vi "app - monitor RUS scan - P1.vi"() -> ()   [LabVIEW 2014]
uses:
  complex region.ctl
  lorentzian.ctl
  circle corners.ctl
  cursor winow.ctl
  scale - offset gauge.ctl
  <vilib>/event_ctls.llb/eventvkey.ctl
  peak -- parameters -- complex fit.ctl
  wavepacket.ctl
  filter method control.ctl
  parameters -- scan monitor control.ctl
  monitor state.ctl
  peak monitor ctl.ctl
  interpolation state - real.ctl
  countdown control.ctl
  cursor window action.ctl
  plot refs -- filter related.ctl
  monitor action.ctl
  read scan file control.ctl
  ctl -- name dispatcher -- action.ctl
  Q -- check range -- i -- real - window.vi
  array -- find interval - real.vi
  next chunk - read-write freq PID file - atomic actions .vi
  Q -- check range -- i -- integer.vi
  aggregator - iii - real - atomic.vi
  switch - C.vi
  acquire cursor window data.vi
  filter - complex - four.vi
  peak -- PM find lorenzian - V2.vi
  Q - not nan -- real.vi
  array -- find index - real.vi
  array -- interpolate -- i.vi
  Q - not nan -- integer.vi
  linear interpolation - real.vi
  tale of three indices.vi
  filter -- window span logic.vi
  linear interp iiii- complex - z-omega - divide.vi
  linear interpolation iiii- complex.vi
  containing bix.vi
  peak -- guess at omega -- dzdomega.vi
  command stack.vi
  tale of three indices -- check state.vi
  linear interp iiii- complex - z-omega.vi
  line -- complex.vi
  peak -- z center from mult phase points.vi
  peak -- estimate for lorentzian.vi
  peak -- fake phase around center.vi
  peak -- get weights.vi
  peak -- four corner circle transformation logic.vi
  peak - fit phase around center - V1.vi
  <vilib>/Analysis/baseanly.llb/A x B.vi
  <vilib>/Analysis/baseanly.llb/Complex A x B.vi
  circle center from three points.vi
  <vilib>/Utility/error.llb/Clear Errors.vi
  Split file name.vi
  <vilib>/Utility/file.llb/Read From Spreadsheet File.vi
  <vilib>/Utility/file.llb/Read From Spreadsheet File (DBL).vi
  <vilib>/Utility/file.llb/Read From Spreadsheet File (string).vi
  Q regex box.vi
  <vilib>/Utility/libraryn.llb/Check if File or Folder Exists.vi
  file -- read list of lines.vi
  parse -- find first line.vi
  parse -- get list of matches -- numbers.vi
  <vilib>/Utility/file.llb/Write To Spreadsheet File (string).vi
  <vilib>/gmath/function.llb/Binomial Coefficient.vi
  monitor -- write section files.vi
  <vilib>/Analysis/Matrix/Numeric/Conversions/Array To Matrix.vi
  <vilib>/Analysis/Matrix/Numeric/Conversions/Array To Matrix - RA2.vi
  <vilib>/Analysis/baseanly.llb/Inverse Matrix.vi
  <vilib>/Analysis/baseanly.llb/Real Inverse Matrix.vi
  array - generate range.vi
  peak -- fit function -- arctan.vi
  <vilib>/gmath/NumericalOptimization/Nonlinear Curve Fit.vi
  <vilib>/gmath/NumericalOptimization/Nonlinear Curve Fit LM.vi
  filter pipe - plot staff - more - V2.vi
panel:
  in  "overwriting !!":bool
  in  "current resonance #":i32=2
  in  "overwrite (d)":enum16{"DUMP", "WORK", ""}(ring)
  in  "Tab : monitor":enum32{"main", "EDIT"}(tab)
  out "index -- main":i32[](array[numeric])=[0, 1, 2, 3, 4, 5, 6, 7, 8, 9, 10, 11, 12, 13, 14, 15, 16, 17, 18, 19, 20, 21, 22, 23, 24, 25, 26, 27, 28, 29, 30, 31, 32, 33, 34, 35, 36, 37, 38, 39, 40, 41, 42, 43, 44, 45, 46, 47, 48, 49, 50, 51, 52, 53, 54, 55, 56, 57, 58, 59, 60, 61, 62, 63, 64, 65, 66, 67, 68, 69, 70, 71, 72, 73, 74, 75, 76, 77, 78, 79, 80, 81, 82, 83, 84, 85, 86, 87, 88, 89, 90, 91, 92, 93, 94, 95, 96, 97, 98, 99]
  in  "scan monitor control":T1={"gamma acc. - min "=0.3, "gamma acc. - max"=3.0, "peak acc. fraction"=4.0, "min peak acc. window (kHz)"=0.5, "use"=enum."fraction", "abs gamma min(kHz)"=0.01, "abs gamma max(kHz)"=10.0, "# points"=10, "gamma-factor"=4.0, "interpolate"=enum."line", "init"=TRUE, "Unique peak \nparameters"=FALSE, "max peak acc. window (kHz)"=15.0, "spacing factor"=1.5, "iterate #"=1, "overwrite?"=TRUE, "write \nm files?"=TRUE, "max slope"=0.5}
  in  "monitor state":T2={"header - gamma"=[], "header - frequency"=[], "# of peaks"=6, "peaks OK"=FALSE}
  in  "autopilot":enum32{"on", "off"}(tab)=enum."off"
  in  "\"o\" timer selector":enum32{"absol", "watch"}(tab)=enum."watch"
  in  "timer \"o\"":dbl(slide)=156.2819999998901 min=-451299679.0000001 max=2129711151.0 step=0.010000000000000002 scale=0.0..320.0 scale format="%#3_3f"
  in  "timer  \"update\"":dbl(slide)=6.281999999890104 min=-451449679.0000001 max=2129711151.0 step=0.010000000000000002 scale=0.0..10.0 scale format="%#3_3f"
  in  "timer \"v\"":dbl(slide)=1.2710000000079162 min=-451454690.0 max=2129711151.0 step=0.01 scale=0.0..5.0 scale format="%#3_3f"
  in  "Temperature (K)":dbl=46.363
  in  "Magn Field (T)":dbl
  in  "Array of states":T3[](array[typedef])=[{"delta"=30.039245391659023, "gamma"=0.02588, "exp"=212.58431, "found?"=FALSE, "found"=242.623555391659, "gamma found"=8.56555840842866e-05, "init linear"=TRUE, "interpolate"=enum."line", "gamma-factor"=4.0, "slope"=0.0, "update freq?"=TRUE, "update gamma?"=FALSE, "acc factor"=4.0, "linear interpolation state"={"requested size"=10, "Array"=[0.0, 0.0, 0.0, 0.0, 0.0, 0.0, 0.0, 0.0, 0.0, 212.58431], "actual number of elements"=1}}, {"delta"=0.058120035166581374, "gamma"=0.02588, "exp"=200.03416, "found?"=FALSE, "found"=200.0922800351666, "gamma found"=0.029880221491734887, "init linear"=TRUE, "interpolate"=enum."line", "gamma-factor"=4.0, "slope"=0.0, "update freq?"=TRUE, "update gamma?"=FALSE, "acc factor"=4.0, "linear interpolation state"={"requested size"=10, "Array"=[0.0, 0.0, 0.0, 0.0, 0.0, 0.0, 0.0, 0.0, 0.0, 200.03416], "actual number of elements"=1}}, {"delta"=-414.585032797282, "gamma"=10.0, "exp"=521.21905, "found?"=FALSE, "found"=106.63401720271804, "gamma found"=859.856632431685, "init linear"=FALSE, "interpolate"=enum."line", "gamma-factor"=4.0, "slope"=0.2048099999999712, "update freq?"=TRUE, "update gamma?"=TRUE, "acc factor"=4.0, "linear interpolation state"={"requested size"=10, "Array"=[523.06234, 522.85753, 522.65272, 522.44791, 522.2431, 522.03829, 521.83348, 521.62867, 521.42386, 521.21905], "actual number of elements"=10}}, {"delta"=-82.56675261318571, "gamma"=10.0, "exp"=900.77722, "found?"=FALSE, "found"=818.2104673868143, "gamma found"=202.9884321626993, "init linear"=TRUE, "interpolate"=enum."line", "gamma-factor"=4.0, "slope"=0.0, "update freq?"=TRUE, "update gamma?"=FALSE, "acc factor"=4.0, "linear interpolation state"={"requested size"=10, "Array"=[0.0, 0.0, 0.0, 0.0, 0.0, 0.0, 0.0, 0.0, 0.0, 900.77722], "actual number of elements"=1}}, {"delta"=-2808.68343, "gamma"=0.01, "exp"=2808.68343, "found?"=FALSE, "found"=0.0, "gamma found"=0.0, "init linear"=TRUE, "interpolate"=enum."line", "gamma-factor"=2.0, "slope"=0.0, "update freq?"=TRUE, "update gamma?"=FALSE, "acc factor"=2.0, "linear interpolation state"={"requested size"=10, "Array"=[0.0, 0.0, 0.0, 0.0, 0.0, 0.0, 0.0, 0.0, 0.0, 2808.68343], "actual number of elements"=1}}, {"delta"=115.97601993996977, "gamma"=10.0, "exp"=2981.49794, "found?"=FALSE, "found"=3097.47395993997, "gamma found"=145.01354836282937, "init linear"=TRUE, "interpolate"=enum."line", "gamma-factor"=6.0, "slope"=0.0, "update freq?"=TRUE, "update gamma?"=FALSE, "acc factor"=6.0, "linear interpolation state"={"requested size"=10, "Array"=[0.0, 0.0, 0.0, 0.0, 0.0, 0.0, 0.0, 0.0, 0.0, 2981.49794], "actual number of elements"=1}}]
  in  "dump/work NEW (\"n\")":enum16{"DUMP", "WORK", ""}(ring)
  in  "NEW freq":dbl[](array[numeric])=[212.58431, 200.03416, 521.01424, 900.77722, 2808.68343, 2981.49794]
  in  "NEW gamma":dbl[](array[numeric])=[0.02588, 0.02588, 10.0, 10.0, 0.01, 10.0]
  in  "OLD gamma":dbl[](array[numeric])=[0.02588, 0.02588, 10.0, 10.0, 0.01, 10.0]
  in  "OLD freq":dbl[](array[numeric])=[212.58431, 200.03416, 521.21905, 900.77722, 2808.68343, 2981.49794]
  out "cp lorentzian":T5={"Amplitude"=0.04556963061640163, "omega(0)"=3097.47395993997, "Gamma"=145.01354836282937, "phase"=-0.8570973522961745, "Q"=21.359893574840147, "Norm  Ampl"=nan, "z (inf)"=0.0028057937941274873+0.005057236434013693i, "4corners"={"z (-pi/2)"=0.002773957390370687+0.0046139701857242825i, "z(inf)"=0.0028057937941274873+0.005057236434013693i, "z (pi/2)"=0.0023625275458380767+0.005089072837770493i, "z center"=0.0025682424681043817+0.004851521511747388i, "z(0)"=0.002330691142081276+0.004645806589481083i, "radius"=0.0003142439525883794}} {"z (inf)" format="%#9_9f"; "Q" format="%#9_9f"; "phase" format="%#9_9f"; "Gamma" format="%#9_9f"; "omega(0)" format="%#9_9f"}
  out "index":i32[](array[numeric])=[0, 1, 2, 3, 4, 5, 6, 7, 8, 9, 10, 11, 12, 13, 14, 15, 16, 17, 18, 19, 20, 21, 22, 23, 24, 25, 26, 27, 28, 29, 30, 31, 32, 33, 34, 35, 36, 37, 38, 39, 40, 41, 42, 43, 44, 45, 46, 47, 48, 49, 50, 51, 52, 53, 54, 55, 56, 57, 58, 59, 60, 61, 62, 63, 64, 65, 66, 67, 68, 69, 70, 71, 72, 73, 74, 75, 76, 77, 78, 79, 80, 81, 82, 83, 84, 85, 86, 87, 88, 89, 90, 91, 92, 93, 94, 95, 96, 97, 98, 99]
  in  "Tab : everything":T7(tab)
  in  "Tab :  Fit controls":enum32{"complex plane", "complex plane 2"}(tab)
  in  "Plot: fragment - filter":cluster{dbl[], dbl[]}[](graph)=[{array[466 elements], array[466 elements]}, {array[466 elements], array[466 elements]}, {array[466 elements], array[466 elements]}, {array[466 elements], array[466 elements]}]
  in  "scale gauge: Plot: complex plane - filter":dbl(slide)=0.001 min=0.0 max=0.3 step=1e-05 scale=0.0001..0.3 scale format="%#_2g"
  in  "Plot: complex plane - filter":cluster{dbl[], dbl[]}[](graph)=[{array[466 elements], array[466 elements]}, {array[466 elements], array[466 elements]}, {[0.009289136459626816, 0.00928889692413463, 0.009288179262995223, 0.009286986308489249, 0.009285322768663132, 0.009283195208748563, 0.00928061202525254, 0.009277583412820176, 0.0092741213240011, 0.009270239422078202, 0.0092659530271449, 0.009261279055643728, 0.009256235953604868, 0.009250843623848093, 0.009245123347435429, 0.009239097699684534, 0.009232790461074223, 0.009226226523393789, 0.009219431791506477, 0.00921243308111483, 0.009205258012931357, 0.0091979349036722, 0.009190492654303994, 0.009182960635984958, 0.009175368574150343, 0.009167746431199728, 0.009160124288249112, 0.009152532226414498, 0.009145000208095461, 0.009137557958727257, 0.0091302348494681, 0.009123059781284627, 0.009116061070892979, 0.009109266339005667, 0.009102702401325232, 0.009096395162714922, 0.009090369514964027, 0.009084649238551363, 0.009079256908794587, 0.009074213806755728, 0.009069539835254556, 0.009065253440321254, 0.009061371538398356, 0.00905790944957928, 0.009054880837146916, 0.009052297653650893, 0.009050170093736324, 0.009048506553910207, 0.009047313599404232, 0.009046595938264826, 0.00904635640277264, 0.009046595938264826, 0.009047313599404232, 0.009048506553910207, 0.009050170093736324, 0.009052297653650893, 0.009054880837146916, 0.00905790944957928, 0.009061371538398356, 0.009065253440321254, 0.009069539835254556, 0.009074213806755728, 0.009079256908794587, 0.009084649238551363, 0.009090369514964027, 0.009096395162714922, 0.009102702401325232, 0.009109266339005667, 0.009116061070892979, 0.009123059781284627, 0.0091302348494681, 0.009137557958727257, 0.009145000208095461, 0.009152532226414498, 0.009160124288249112, 0.009167746431199728, 0.009175368574150343, 0.009182960635984958, 0.009190492654303994, 0.0091979349036722, 0.009205258012931357, 0.00921243308111483, 0.009219431791506477, 0.009226226523393789, 0.009232790461074223, 0.009239097699684534, 0.009245123347435429, 0.009250843623848093, 0.009256235953604868, 0.009261279055643728, 0.0092659530271449, 0.009270239422078202, 0.0092741213240011, 0.009277583412820176, 0.00928061202525254, 0.009283195208748563, 0.009285322768663132, 0.009286986308489249, 0.009288179262995223, 0.00928889692413463], [0.002651237221672282, 0.002658859364622897, 0.002666451426457512, 0.002673983444776548, 0.002681425694144753, 0.00268874880340391, 0.002695923871587384, 0.0027029225819790313, 0.002709717313866343, 0.002716281251546778, 0.0027225884901570883, 0.002728614137907983, 0.002734334414320646, 0.002739726744077422, 0.0027447698461162827, 0.002749443817617454, 0.0027537302125507554, 0.0027576121144736536, 0.00276107420329273, 0.0027641028157250947, 0.002766685999221118, 0.002768813559135685, 0.0027704770989618035, 0.0027716700534677783, 0.002772387714607183, 0.0027726272500993698, 0.002772387714607183, 0.0027716700534677783, 0.0027704770989618035, 0.002768813559135685, 0.002766685999221118, 0.0027641028157250947, 0.00276107420329273, 0.0027576121144736536, 0.0027537302125507554, 0.002749443817617454, 0.0027447698461162827, 0.002739726744077422, 0.002734334414320646, 0.002728614137907983, 0.0027225884901570883, 0.002716281251546778, 0.002709717313866343, 0.0027029225819790313, 0.002695923871587384, 0.00268874880340391, 0.002681425694144753, 0.002673983444776548, 0.0026664514264575115, 0.002658859364622897, 0.002651237221672282, 0.002643615078721667, 0.002636023016887052, 0.002628490998568016, 0.002621048749199811, 0.0026137256399406538, 0.00260655057175718, 0.0025995518613655326, 0.002592757129478221, 0.002586193191797786, 0.0025798859531874756, 0.002573860305436581, 0.002568140029023918, 0.002562747699267142, 0.002557704597228281, 0.00255303062572711, 0.002548744230793808, 0.0025448623288709103, 0.0025414002400518335, 0.002538371627619469, 0.002535788444123446, 0.002533660884208879, 0.0025319973443827604, 0.0025308043898767856, 0.0025300867287373807, 0.002529847193245194, 0.0025300867287373807, 0.0025308043898767856, 0.0025319973443827604, 0.002533660884208879, 0.002535788444123446, 0.002538371627619469, 0.002541400240051834, 0.0025448623288709103, 0.0025487442307938085, 0.00255303062572711, 0.002557704597228281, 0.002562747699267142, 0.002568140029023918, 0.002573860305436581, 0.0025798859531874756, 0.002586193191797786, 0.002592757129478221, 0.0025995518613655326, 0.00260655057175718, 0.0026137256399406538, 0.002621048749199811, 0.002628490998568016, 0.0026360230168870524, 0.002643615078721667]}, {[-8.885828284567812e-06, -1.4167771767865586e-05, -2.3057643869771674e-05], [8.639843856131629e-06, -5.498795551443347e-06, 3.022123088162283e-05]}, {[-1.3695780266495954e-05, -1.2414352587154252e-05, -1.1132924907812547e-05, -9.851497228470845e-06, -8.570069549129142e-06, -7.288641869787439e-06, -6.007214190445735e-06, -4.725786511104032e-06, -3.4443588317623295e-06, -2.162931152420627e-06, -8.815034730789241e-07, 3.9992420626278023e-07, 1.6813518856044846e-06, 2.9627795649461873e-06, 4.24420724428789e-06, 5.525634923629593e-06, 6.807062602971295e-06, 8.088490282312998e-06, 9.3699179616547e-06, 1.0651345640996403e-05], [-2.395985450805763e-05, -2.3725197032175156e-05, -2.3490539556292678e-05, -2.3255882080410203e-05, -2.3021224604527724e-05, -2.278656712864525e-05, -2.2551909652762774e-05, -2.2317252176880296e-05, -2.208259470099782e-05, -2.1847937225115342e-05, -2.1613279749232868e-05, -2.1378622273350393e-05, -2.1143964797467914e-05, -2.090930732158544e-05, -2.067464984570296e-05, -2.0439992369820486e-05, -2.020533489393801e-05, -1.9970677418055532e-05, -1.9736019942173057e-05, -1.950136246629058e-05]}, {[-1.4167771767865586e-05, -1.2116340982462017e-05, -1.0064910197058446e-05, -8.013479411654875e-06, -5.962048626251305e-06, -3.910617840847736e-06, -1.8591870554441647e-06, 1.9224372995940643e-07, 2.243674515362976e-06, 4.295105300766545e-06, 6.346536086170115e-06, 8.397966871573687e-06, 1.0449397656977257e-05, 1.2500828442380826e-05, 1.4552259227784399e-05, 1.660369001318797e-05, 1.8655120798591538e-05, 2.0706551583995107e-05, 2.2757982369398677e-05, 2.4809413154802246e-05], [-5.498795551443347e-06, -5.498795551443347e-06, -5.498795551443347e-06, -5.498795551443347e-06, -5.498795551443347e-06, -5.498795551443347e-06, -5.498795551443347e-06, -5.498795551443347e-06, -5.498795551443347e-06, -5.498795551443347e-06, -5.498795551443347e-06, -5.498795551443347e-06, -5.498795551443347e-06, -5.498795551443347e-06, -5.498795551443347e-06, -5.498795551443347e-06, -5.498795551443347e-06, -5.498795551443347e-06, -5.498795551443347e-06, -5.498795551443347e-06]}]
  out "Plot: dz/domega":cluster{"omega out":dbl[], dbl[]}(graph)
  out "Plot: win omega":T8(graph)
  out "Plot: phase":cluster{"omega out":dbl[], dbl[]}(graph)
  out "Plot: phase around center":cluster{dbl[], dbl[]}[](graph)
  out "Plot: fragment":cluster{dbl[], dbl[]}[](graph)
  out "Plot: complex plane":cluster{dbl[], dbl[]}[](graph)=[{array[466 elements], array[466 elements]}, {[0.009207737399172267, 0.009207524932737727, 0.0092068908841567, 0.009205845252754072, 0.009204404528761694, 0.009202591433257568, 0.00920043455984089, 0.00919796792369389, 0.009195230425142106, 0.009192265236173003, 0.009189119119587938, 0.00918584169152486, 0.009182484638982163, 0.009179100904683851, 0.009175743852141155, 0.009172466424078077, 0.009169320307493012, 0.009166355118523909, 0.009163617619972125, 0.009161150983825125, 0.009158994110408446, 0.009157181014904321, 0.009155740290911943, 0.009154694659509315, 0.009154060610928287, 0.009153848144493748, 0.009154060610928287, 0.009154694659509315, 0.009155740290911943, 0.009157181014904321, 0.009158994110408446, 0.009161150983825125, 0.009163617619972125, 0.009166355118523909, 0.009169320307493012, 0.009172466424078077, 0.009175743852141155, 0.009179100904683851, 0.009182484638982163, 0.00918584169152486, 0.009189119119587938, 0.009192265236173003, 0.009195230425142106, 0.00919796792369389, 0.00920043455984089, 0.009202591433257568, 0.009204404528761694, 0.009205845252754072, 0.0092068908841567, 0.009207524932737727], [0.002661906885220897, 0.0026652839424925116, 0.0026686077415535962, 0.002671825864107417, 0.0026748875584388866, 0.00267774453979943, 0.0026803517518863137, 0.0026826680774074546, 0.0026846569865256785, 0.002686287112956074, 0.002687532748631044, 0.002688374249131887, 0.0026887983434930166, 0.0026887983434930166, 0.002688374249131887, 0.002687532748631044, 0.002686287112956074, 0.0026846569865256785, 0.0026826680774074546, 0.0026803517518863137, 0.00267774453979943, 0.0026748875584388866, 0.002671825864107417, 0.0026686077415535962, 0.0026652839424925116, 0.002661906885220897, 0.0026585298279492822, 0.0026552060288881976, 0.0026519879063343767, 0.002648926212002907, 0.0026460692306423637, 0.00264346201855548, 0.0026411456930343392, 0.0026391567839161153, 0.00263752665748572, 0.0026362810218107497, 0.002635439521309907, 0.002635015426948777, 0.002635015426948777, 0.002635439521309907, 0.0026362810218107497, 0.00263752665748572, 0.0026391567839161153, 0.0026411456930343392, 0.00264346201855548, 0.0026460692306423637, 0.002648926212002907, 0.0026519879063343767, 0.0026552060288881976, 0.0026585298279492822]}, {[0.009205382317068227, 0.009202923362544706, 0.009200464408021183, 0.009198005453497662, 0.009195546498974139, 0.009193087544450617, 0.009190628589927096, 0.009188169635403573, 0.009185710680880052, 0.009183251726356529, 0.009180792771833007, 0.009178333817309486, 0.009175874862785963, 0.009173415908262442, 0.009170956953738919, 0.009168497999215397, 0.009166039044691876, 0.009163580090168353, 0.009161121135644832, 0.009158662181121309], [0.0026508902066117793, 0.002651991874472691, 0.002653093542333603, 0.0026541952101945144, 0.0026552968780554262, 0.002656398545916338, 0.00265750021377725, 0.002658601881638162, 0.0026597035494990732, 0.002660805217359985, 0.002661906885220897, 0.0026630085530818088, 0.0026641102209427206, 0.002665211888803632, 0.002666313556664544, 0.0026674152245254558, 0.0026685168923863676, 0.0026696185602472795, 0.002670720228108191, 0.0026718218959691027]}, {[0.00916977609322389, 0.009170877761084802, 0.009171979428945713, 0.009173081096806625, 0.009174182764667537, 0.00917528443252845, 0.00917638610038936, 0.009177487768250272, 0.009178589436111185, 0.009179691103972095, 0.009180792771833007, 0.00918189443969392, 0.00918299610755483, 0.009184097775415742, 0.009185199443276655, 0.009186301111137565, 0.009187402778998478, 0.00918850444685939, 0.009189606114720302, 0.009190707782581213], [0.002637317339985676, 0.002639776294509198, 0.0026422352490327204, 0.002644694203556242, 0.0026471531580797643, 0.0026496121126032865, 0.0026520710671268087, 0.002654530021650331, 0.0026569889761738526, 0.0026594479306973747, 0.002661906885220897, 0.002664365839744419, 0.0026668247942679413, 0.002669283748791463, 0.002671742703314985, 0.0026742016578385074, 0.0026766606123620296, 0.0026791195668855517, 0.0026815785214090735, 0.0026840374759325956]}, {[-0.08465297135149538, -0.08709700955873212, -0.08948087657263201, -0.0918030825539097, -0.09406217619941787, -0.09625674564916473, -0.09838541936868056, -0.10044686700618197, -0.10243980022399857, -0.10436297350374193, -0.10621518492471424, -0.1079952769150695, -0.10970213697525821, -0.11133469837330345, -0.11289194081147358, -0.11437289106393522, -0.11577662358498755, -0.11710226108749844, -0.11834897509118011, -0.1195159864403626], [0.10160144570548792, 0.09922489930928838, 0.09678800095446072, 0.09429227362315218, 0.09173927706370548, 0.08913060681586663, 0.08646789321362464, 0.08375280036630582, 0.08098702511855962, 0.07817229598988612, 0.0753103720943673, 0.0724030420412782, 0.06945212281726429, 0.06645945865078412, 0.06342691985952623, 0.060356401681521774, 0.05724982309068233, 0.05410912559750363, 0.050936272035684876, 0.04773324533542133]}, {[-0.09841542123281663, -0.10121791837711472, -0.10395141921971995, -0.10661421541158506, -0.10920464279176773, -0.11172108242747747, -0.11416196162585562, -0.11652575491685721, -0.11881098500662027, -0.12101622370072598, -0.12314009279677424, -0.1251812649457149, -0.12713846448139798, -0.12901046821782317, -0.1307961062135916, -0.13249426250308094, -0.13410387579388763, -0.13562394013010012, -0.13705350552098844, -0.13839167853471768], [0.11611333645976667, 0.11338822992545786, 0.11059391981192214, 0.10773215247202167, 0.10480471641718947, 0.10181344119966758, 0.09876019626909677, 0.09564688980417119, 0.0924754675200889, 0.08924791145254327, 0.08596623871901503, 0.08263250025813954, 0.07924877954793691, 0.0758171913037063, 0.07233988015639725, 0.06881901931228548, 0.0652568091947896, 0.061655476069278015, 0.05801727065172584, 0.05434446670209031]}, {array[466 elements], array[466 elements]}]
  in  "scale gauge: Plot: complex plane":dbl(slide)=0.00559 min=0.0 max=0.3 step=1e-05 scale=0.0001..0.3 scale format="%#_2g"
  in  "plot staff":enum16{"plot", "do not plot", "a"}(ring)=enum."do not plot"
  out "pm lorentzian":T5={"Amplitude"=0.04556963061640163, "omega(0)"=3097.47395993997, "Gamma"=145.01354836282937, "phase"=-0.8570973522961745, "Q"=21.359893574840147, "Norm  Ampl"=nan, "z (inf)"=0.0028057937941274873+0.005057236434013693i, "4corners"={"z (-pi/2)"=0.002773957390370687+0.0046139701857242825i, "z(inf)"=0.0028057937941274873+0.005057236434013693i, "z (pi/2)"=0.0023625275458380767+0.005089072837770493i, "z center"=0.0025682424681043817+0.004851521511747388i, "z(0)"=0.002330691142081276+0.004645806589481083i, "radius"=0.0003142439525883794}} {"z (inf)" format="%#9_9f"; "Q" format="%#9_9f"; "phase" format="%#9_9f"; "Gamma" format="%#9_9f"; "omega(0)" format="%#9_9f"}
  in  "use fast fit?":bool
  out "window width (kHz)":dbl=4.307387926151117
  out "window center (kHz)":dbl=696.64284
  out "# of points in window":dbl=480.8162103439331
  in  "Tab : all plot":enum32{"Page 1"}(tab)
  in  "scale gauge : All plot":T9={"scale offset"=0.5005000000000001, "scale range"=0.019950000000000002} {"scale range" min=0.0 max=1.0 step=1e-05 scale=0.001..1.0 scale format="%#_2g"; "scale offset" min=0.0 max=1.0 step=1e-05 scale=0.001..1.0 scale format="%#_2g"}
  out "Plot: All":cluster{"all rows":dbl[], "all rows":dbl[]}[](graph)
  in  "Sweep folder path":path=path "D:/Technique/RUS/LSCO/LSCO20_131009I/3_warmup1"
  out "scan file found":bool=TRUE
  in  "source":enum16{"last scan file", "manual"}(ring)
  out "complex region":T10={"max re"=1.5, "min re"=-1.5, "max im"=1.5, "min im"=-1.5, "delta re"=3.0, "delta im"=3.0, "center re"=0.0, "delta  z"=3.0+3.0i, "center im"=0.0, "center z"=0.0+0.0i, "d im"=0.0, "d re"=0.0, "d z"=0.0+0.0i}
  in  "cursor bracket: All, data window":T11={"left"=2951.49794, "right "=3011.49794, "center"=2981.49794, "window"=60.0, "cursors"=[0, 1, 2], "relative"=0, "absolute"=0, "fixed vertical offset"=0.0, "vertical offset"=0.0, "skew"=0.0, "default window frac"=0.1, "kind"=enum."symmetric", "skew.left"=0.5, "skew.right"=0.5, "Plot ref"=refnum, "wing order"=enum."back"}
  out "all:min omega":dbl=101.5
  out "all:max omega":dbl=3503.0875055646493
  in  "file path":path=path "D:/Technique/RUS/LSCO/LSCO20_131009I/3_warmup1/July_2015/072515/46.36300K_100_3500_0.50000V_0.00000T_Jul25-2015__17-11-36_001_072515.bin"
  in  "Tab : parameters":enum32{"Page 1"}(tab)
  out "VKey":T12=enum."Down"
  out "Char":i16
  in  "parameters: complex fit":T13={"main VI path"=path "E:/ProjectLocker/LANL/Libraries/control rus sweep -- library/monitor RUS scan.vi", "scale factor"=3.0, "# of grid points"=150, "parameters: wavepacket"={"R"=0.5, "wave number"=22.0, "delta k"=7.0, "radii vector"=[], "radial section"=[], "wave vector"=22.0, "wavepacket is"=TRUE}, "span"=0.33799, "interference ?"=enum."pm zcenter", "filter method"=enum."three"} {"span" min=0.0 max=0.5 step=1e-05 scale=0.0001..0.5 scale format="%#_5f"; "parameters: wavepacket"."delta k" format="%#_3f"; "parameters: wavepacket"."wave number" format="%#_3f"; "parameters: wavepacket"."R" format="%#_3f"}
  out "4corners":T6={"z (-pi/2)"=0.006197557655001167-0.00034937824615747343i, "z(inf)"=0.00621689329014135-0.0006376347632966253i, "z (pi/2)"=0.006505149807280503-0.0006182991281564415i, "z center"=0.006351353731140835-0.00048383868715695747i, "z(0)"=0.00648581417214032-0.0003300426110172896i, "radius"=0.0002042861797325857}
  out "good lorentzian":T5={"Amplitude"=9.77117276869725e-06, "omega(0)"=696.6258300994124, "Gamma"=0.3626390020418114, "phase"=4.291180453770643, "Q"=1920.98981680711, "Norm  Ampl"=nan, "z (inf)"=0.009205382317068227+0.0026508902066117793i, "4corners"={"z (-pi/2)"=0.00916977609322389+0.002637317339985676i, "z(inf)"=0.009205382317068227+0.0026508902066117793i, "z (pi/2)"=0.009191809450442125+0.002686496430456118i, "z center"=0.009180792771833007+0.002661906885220897i, "z(0)"=0.009156203226597787+0.0026729235638300146i, "radius"=2.694462733925929e-05}} {"z (inf)" format="%#9_9f"; "Q" format="%#9_9f"; "phase" format="%#9_9f"; "Gamma" format="%#9_9f"; "omega(0)" format="%#9_9f"}
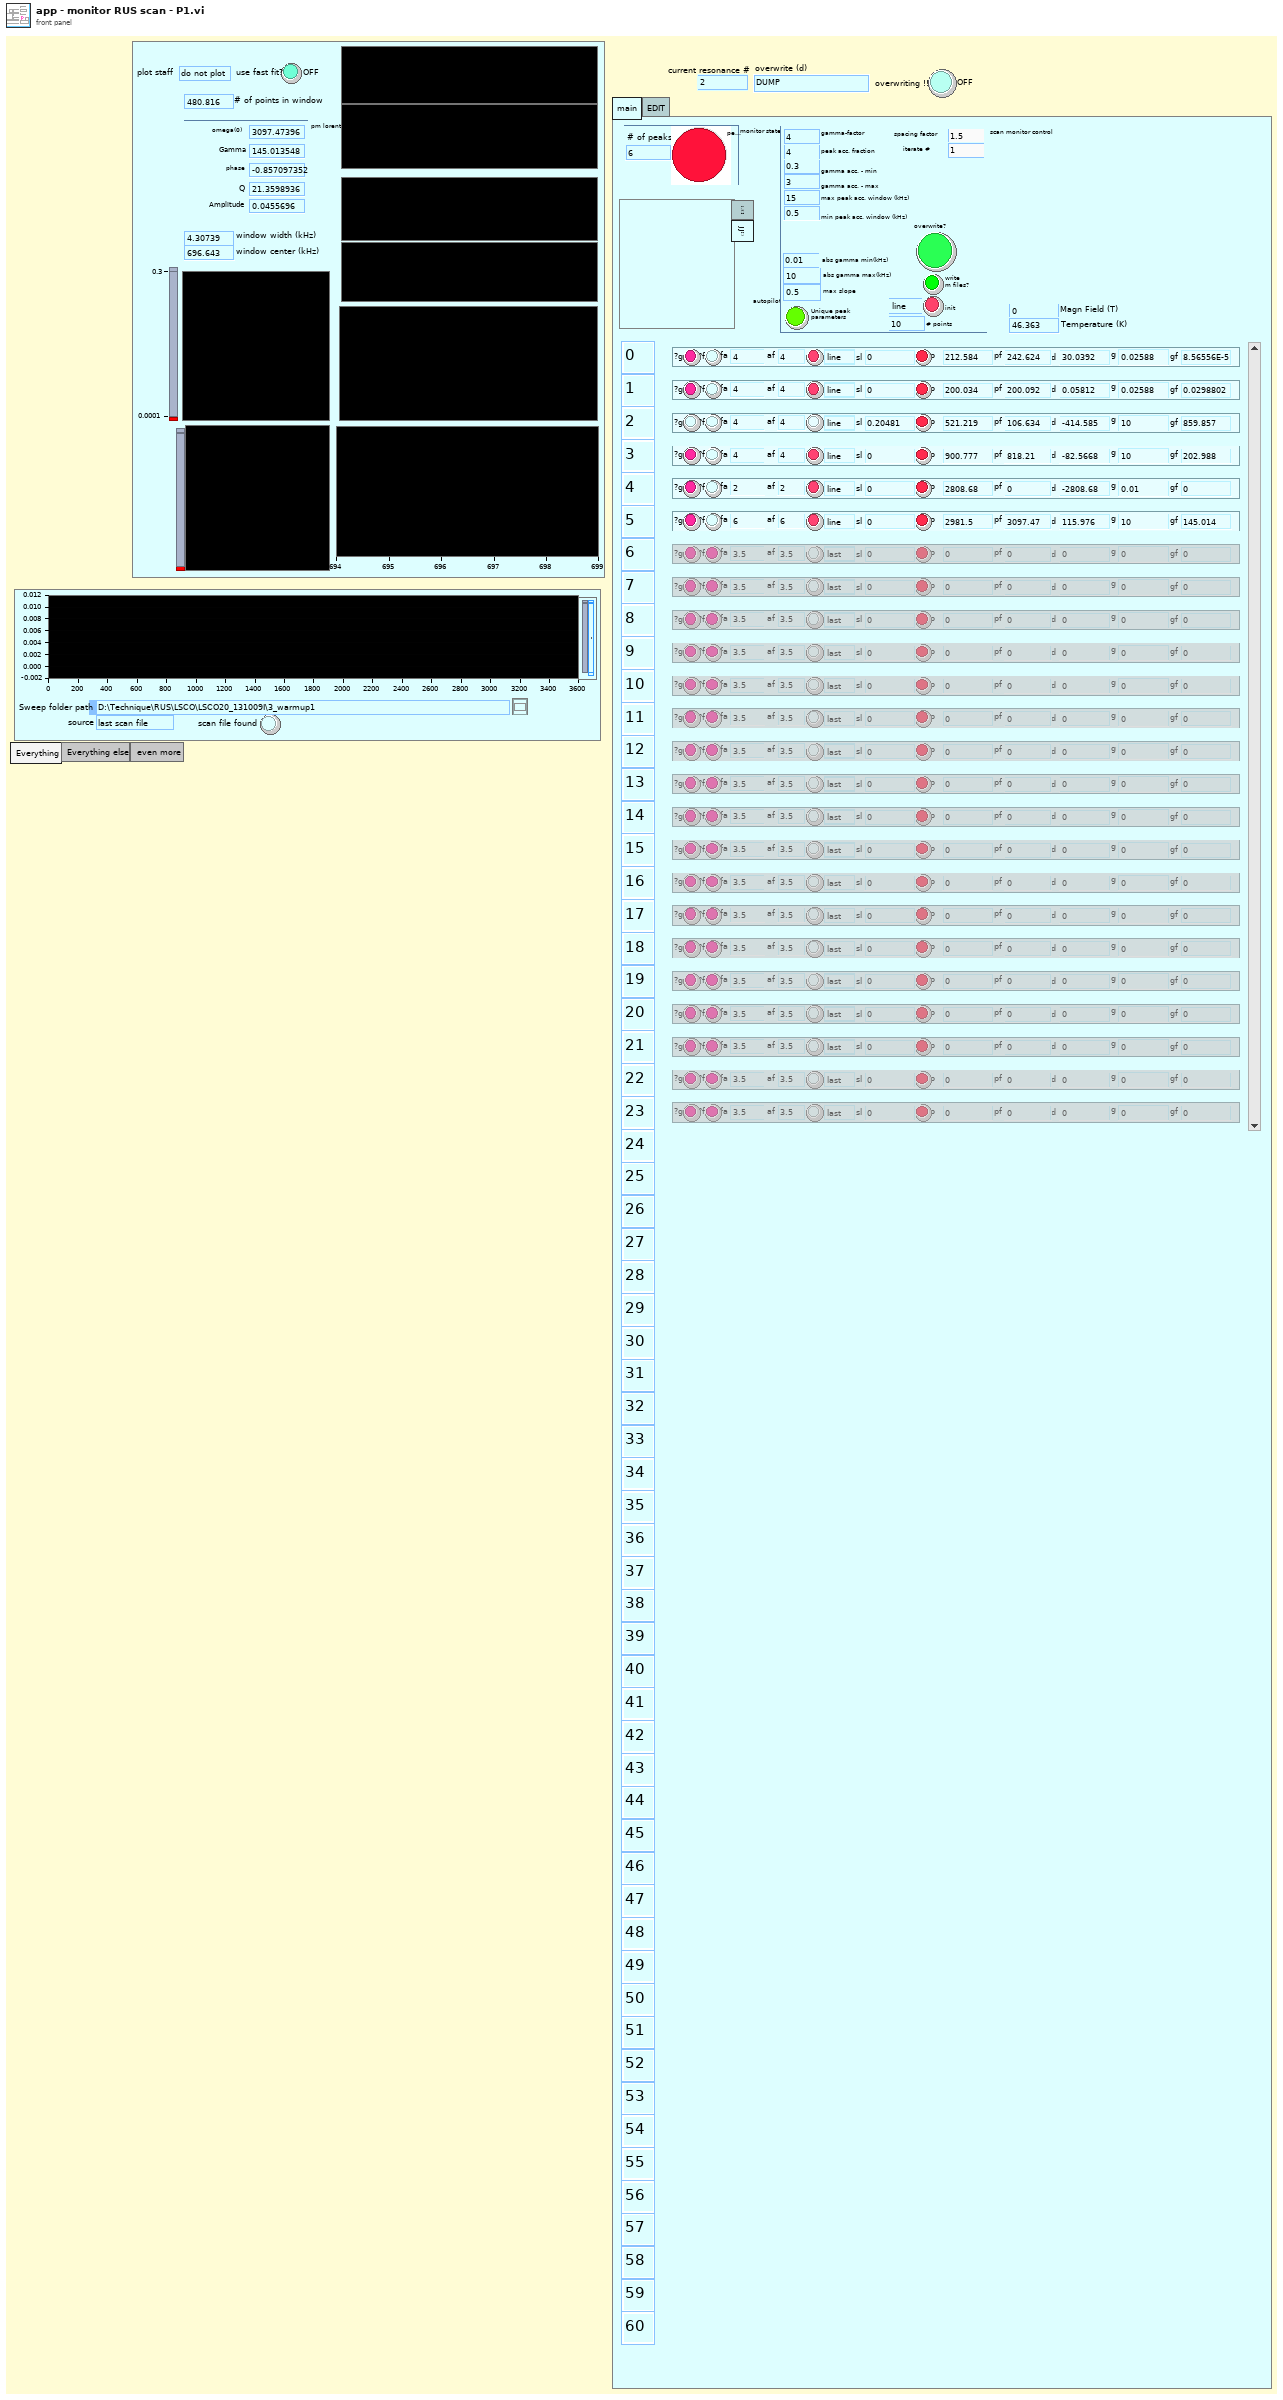
[diagram p1: front panel]
types:
  T1 = typedef "parameters -- scan monitor control.ctl" = cluster{"gamma acc. - min ":dbl, "gamma acc. - max":dbl, "peak acc. fraction":dbl, "min peak acc. window (kHz)":dbl, "use":enum16{"window", "fraction"}, "abs gamma min(kHz)":dbl, "abs gamma max(kHz)":dbl, "# points":i32, "gamma-factor":dbl, "interpolate":enum16{"line", "last"}, "init":bool, "Unique peak \nparameters":bool, "max peak acc. window (kHz)":dbl, "spacing factor":dbl, "iterate #":i32, "overwrite?":bool, "write \nm files?":bool, "max slope":dbl}
  T2 = typedef "monitor state.ctl" = cluster{"header - gamma":string[], "header - frequency":string[], "# of peaks":i32, "peaks OK":bool}
  T3 = typedef "peak monitor ctl.ctl" = cluster{"delta":dbl, "gamma":dbl, "exp":dbl, "found?":bool, "found":dbl, "gamma found":dbl, "init linear":bool, "interpolate":enum16{"line", "last"}, "gamma-factor":dbl, "slope":dbl, "update freq?":bool, "update gamma?":bool, "acc factor":dbl, "linear interpolation state":T4}
  T4 = typedef "interpolation state - real.ctl" = cluster{"requested size":i32, "Array":dbl[], "actual number of elements":i32}
  T5 = typedef "lorentzian.ctl" = cluster{"Amplitude":dbl, "omega(0)":dbl, "Gamma":dbl, "phase":dbl, "Q":dbl, "Norm  Ampl":dbl, "z (inf)":cdb, "4corners":T6}
  T6 = typedef "circle corners.ctl" = cluster{"z (-pi/2)":cdb, "z(inf)":cdb, "z (pi/2)":cdb, "z center":cdb, "z(0)":cdb, "radius":dbl}
  T7 = enum32{"Everything", "Everything else", "even more "}
  T8 = cluster{"omega out":dbl[], "win omega out":dbl[]}
  T9 = typedef "scale - offset gauge.ctl" = cluster{"scale offset":dbl, "scale range":dbl}
  T10 = typedef "complex region.ctl" = cluster{"max re":dbl, "min re":dbl, "max im":dbl, "min im":dbl, "delta re":dbl, "delta im":dbl, "center re":dbl, "delta  z":cdb, "center im":dbl, "center z":cdb, "d im":dbl, "d re":dbl, "d z":cdb}
  T11 = typedef "cursor winow.ctl" = cluster{"left":dbl, "right ":dbl, "center":dbl, "window":dbl, "cursors":i32[], "relative":i32, "absolute":i32, "fixed vertical offset":dbl, "vertical offset":dbl, "skew":dbl, "default window frac":dbl, "kind":enum16{"symmetric", "skewed", "fancy"}, "skew.left":dbl, "skew.right":dbl, "Plot ref":refnum<vi>, "wing order":enum16{"forw", "back"}}
  T12 = typedef "eventvkey.ctl" = enum16{"ASCII", "Enter", "Return", "Shift", "Ctrl", "Alt", "Cmd", "Opt", "Caps", "NumLock", "Clear", "Break", "Up", "Down", "Left", "Right", "Insert", "Delete", "Home", "End", "PageUp", "PageDown", "Escape", "Help", "Pause", "ScrollLock", "F1", "F2", "F3", "F4", "F5", "F6", "F7", "F8", "F9", "F10", "F11", "F12", "F13", "F14", "F15", "F16", "F17", "F18", "F19", "F20", "F21", "F22", "F23", "F24", "Play", "VolumeUp", "VolumeDown", "Mute", "Two Byte Char"}
  T13 = typedef "peak -- parameters -- complex fit.ctl" = cluster{"main VI path":path, "scale factor":dbl, "# of grid points":i32, "parameters: wavepacket":T14, "span":dbl, "interference ?":enum16{"cp z center", "pm zcenter", "fancy"}, "filter method":T15}
  T14 = typedef "wavepacket.ctl" = cluster{"R":dbl, "wave number":dbl, "delta k":dbl, "radii vector":dbl[], "radial section":cdb[], "wave vector":dbl, "wavepacket is":bool}
  T15 = typedef "filter method control.ctl" = enum16{"four", "five", "one", "two", "three", "zero", "minus one", "minus two"}
  T16 = typedef "countdown control.ctl" = enum16{"check", "start", "reset cont", "stop", "reset once"}
  T17 = typedef "plot refs -- filter related.ctl" = cluster{"Plot: complex plane - filter":refnum<vi>, "Plot: dz/domega":refnum<vi>, "Plot: fragment filter":refnum<vi>, "Plot: win omega":refnum<vi>, "Plot: phase":refnum<vi>, "Plot: phase around center":refnum<vi>, "Plot: complex plane":refnum<vi>, "Plot: fragment":refnum<vi>}
  T18 = typedef "cursor window action.ctl" = enum16{"balance", "h. offset change", "cursor moves", "change center", "change window", "init", "check", "reset", "set y to middle", "idle", "-write all Y", "-write left.X", "-write center.X", "-write right.X", "-write all X", "-change center", "-change window", "-change skew", "-read cursor 2", "-read cursor 1", "-read cursor 0", "-read all cursors", "-reset", "-read plot scale", "-set y to middle", "-Q: center.Y is visible", "-Q: window is visible", "-parse center.Y", "-right left from center", "-left move", "-right move", "-set center.Y", "-empty", "-set cursors to default", "-check", "-write center.Y", "-copy cursor 1", "-copy cursor 0", "-copy cursor 2", "move right", "move left", "shrink", "broaden", "skew up", "skew down", "-write plot scale", "zoom X", "change cen&win", "zoom to all data"}
  T19 = typedef "read scan file control.ctl" = cluster{"# columns":i32, "create bin file":bool, "do not filter":bool, "normalize phase":bool, "read freq units":enum16{"kHz", "Hz"}}
  T20 = typedef "monitor action.ctl" = enum16{"monitor", "interpolate", "global", "read", "overwrite", "write m file", "nothing"}
  T21 = typedef "ctl -- name dispatcher -- action.ctl" = enum16{"peak frequency", "peak frequency DUMP", "peak gamma DUMP", "peak gamma", "peak frequency TEST", "peak gamma TEST", "ultrasonic power", "time in gamma", "set temperature ", "set temperature timer", "peak default gamma", "last scan file", "peak freq gamma TEST", "peak NAMES", "errors", "P_I_D", "P", "I", "D", "power vs time", "power vs time TIMER", "void", "power log", "set temperature - SINE", "itc ltc log", "peak - time in gamma"}
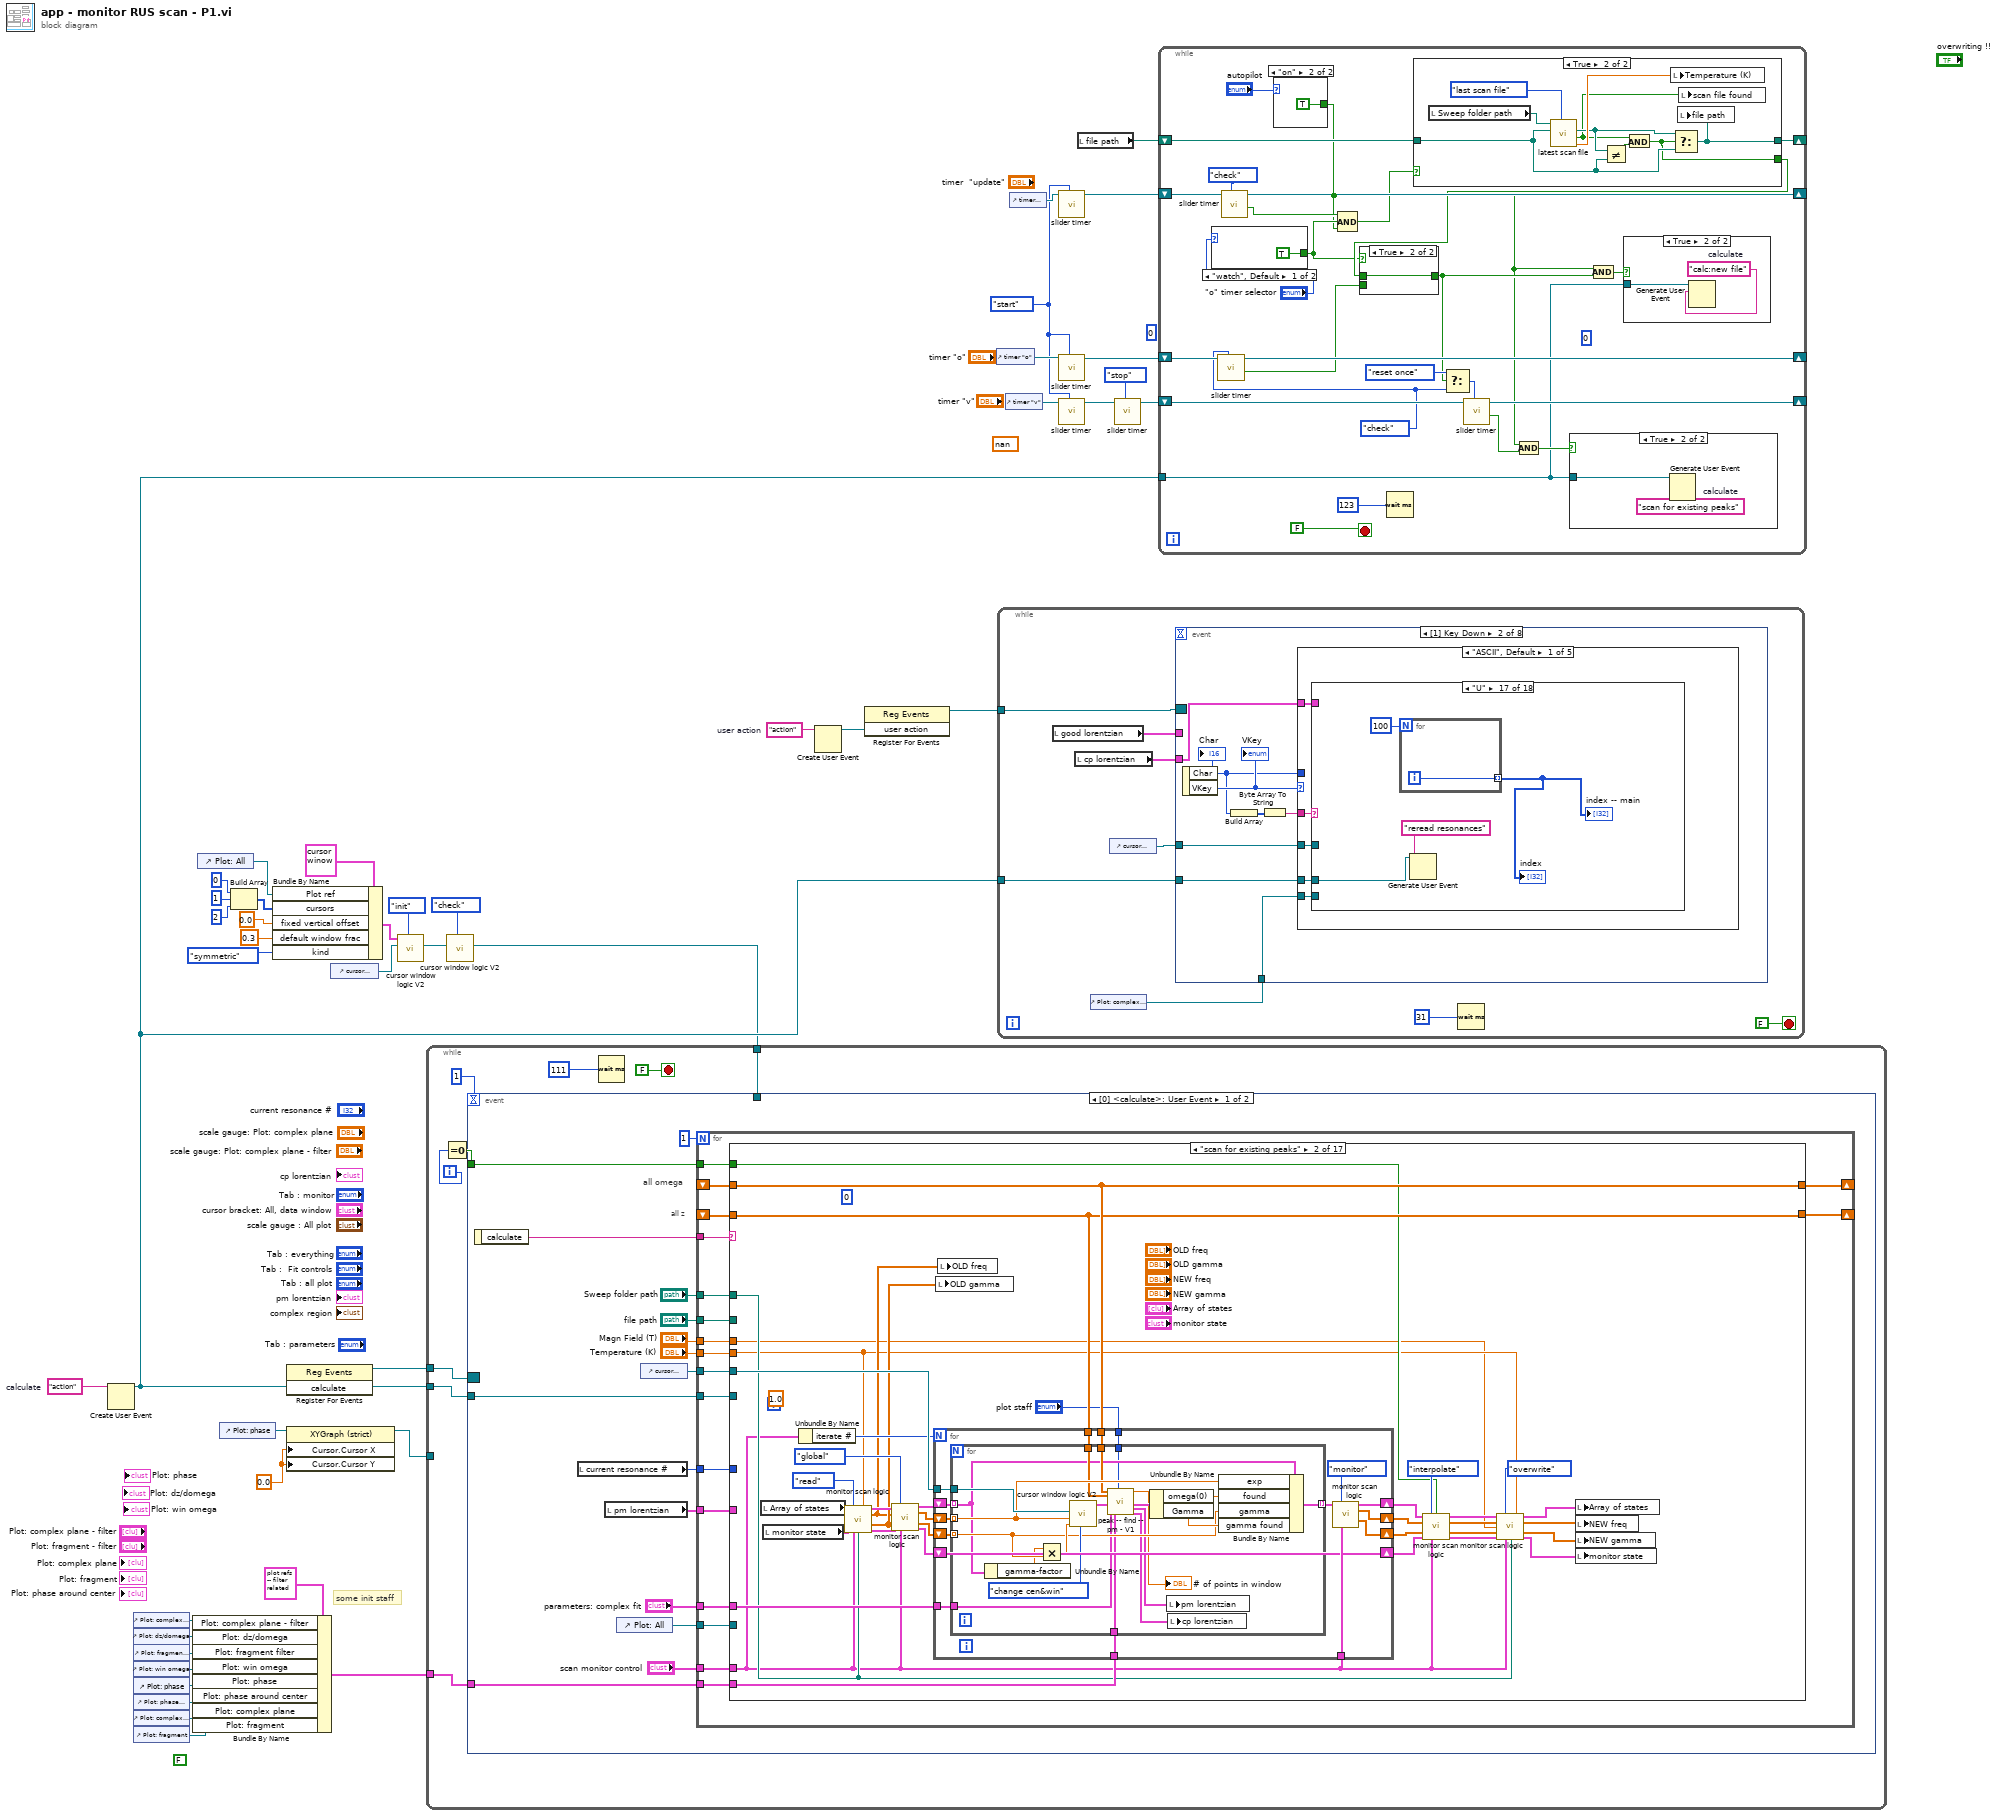
[diagram p0: block diagram]
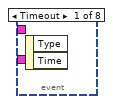
[diagram p2: hidden frame]
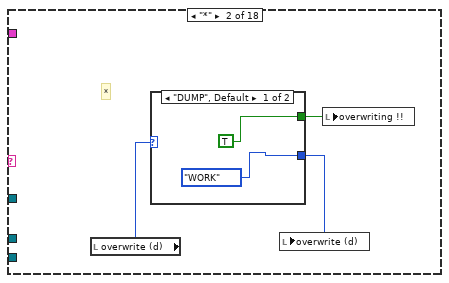
[diagram p4: hidden frame]
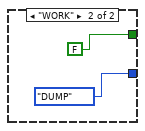
[diagram p5: hidden frame]
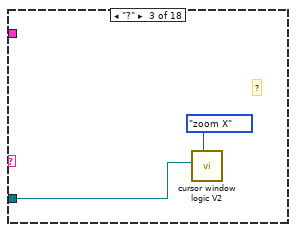
[diagram p6: hidden frame]
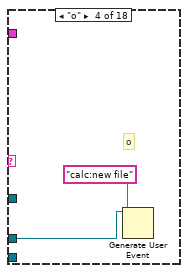
[diagram p7: hidden frame]
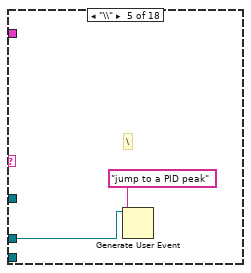
[diagram p8: hidden frame]
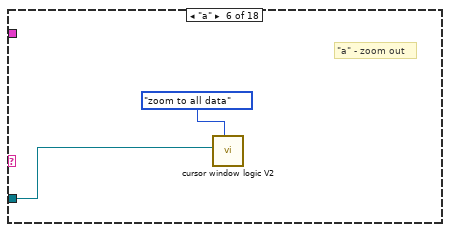
[diagram p9: hidden frame]
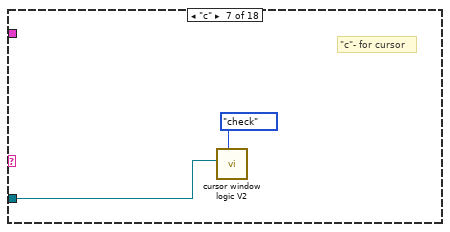
[diagram p10: hidden frame]
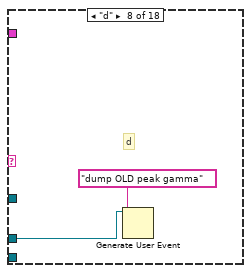
[diagram p11: hidden frame]
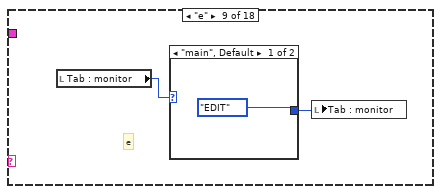
[diagram p12: hidden frame]
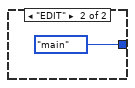
[diagram p13: hidden frame]
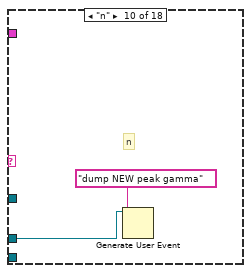
[diagram p14: hidden frame]
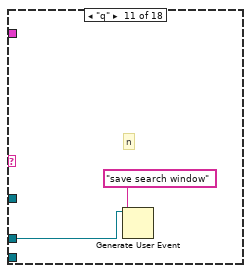
[diagram p15: hidden frame]
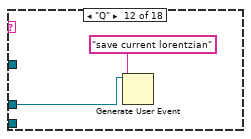
[diagram p16: hidden frame]
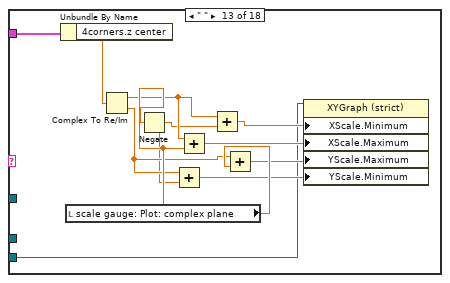
[diagram p17: hidden frame]
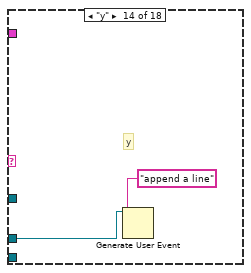
[diagram p18: hidden frame]
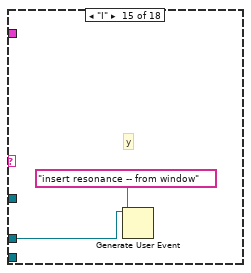
[diagram p19: hidden frame]
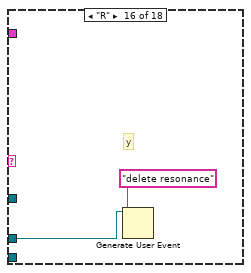
[diagram p20: hidden frame]
diagram:
  (unwired) nan ("\"v\" interval (sec)")
  w19 = 0.0 ("Cursor.Cursor Position:Cursor X")
  w28 = "action"  # user action
  w6 = countdown_control."start" ("action")
  (unwired) 0
  w43 = "action"  # calculate
  (unwired) FALSE
  # "some init staff"
  n1 = Create User Event(user event datatype=w43) -> (user event=w26:refnum<user-event>)  [unwired: 1 in, 1 out]
  n2 = control-ref of="Plot: complex plane - filter"() -> (w16:refnum<vi>)
  n3 = control-ref of="Plot: dz/domega"() -> (w15:refnum<vi>)
  n4 = control-ref of="Plot: fragment - filter"() -> (w14:refnum<vi>)
  n5 = control-ref of="Plot: win omega"() -> (w13:refnum<vi>)
  n6 = control-ref of="Plot: phase"() -> (w12:refnum<vi>)
  n7 = control-ref of="Plot: phase around center"() -> (w10:refnum<vi>)
  n8 = control-ref of="Plot: complex plane"() -> (w9:refnum<vi>)
  n9 = control-ref of="Plot: fragment"() -> (w8:refnum<vi>)
  n10 = Bundle By Name(cluster=T17 {"Plot: complex plane - filter"=refnum, "Plot: dz/domega"=refnum, "Plot: fragment filter"=refnum, "Plot: win omega"=refnum, "Plot: phase"=refnum, "Plot: phase around center"=refnum, "Plot: complex plane"=refnum, "Plot: fragment"=refnum} ("plots: filter related"), "Plot: complex plane - filter"=w16, "Plot: dz/domega"=w15, "Plot: fragment filter"=w14, "Plot: win omega"=w13, "Plot: phase"=w12, "Plot: phase around center"=w10, "Plot: complex plane"=w9, "Plot: fragment"=w8) -> (w11:T17)
  n11 = control-ref of="Plot: All"() -> (w33:refnum<vi>)
  n12 = control-ref of="Plot: phase"() -> (w20:refnum<vi>)
  n13 = Build Array(0, 1, 2) -> (w41:i32[])
  n14 = Bundle By Name(cluster=T11 {"left"=0.0, "right "=0.0, "center"=0.0, "window"=0.0, "cursors"=[], "relative"=0, "absolute"=0, "fixed vertical offset"=0.0, "vertical offset"=0.0, "skew"=0.0, "default window frac"=0.0, "kind"=enum."symmetric", "skew.left"=0.0, "skew.right"=0.0, "Plot ref"=refnum, "wing order"=enum."forw"} ("cursor bracket: All, data window"), "Plot ref"=w33, "cursors"=w41, "fixed vertical offset"=0.0, "default window frac"=0.3 ("fixed vertical offset"), "kind"=enum16{"symmetric", "skewed", "fancy"}."symmetric") -> (w32:T11)
  n15 = register-events(w26) -> (reference out=w44:refnum<event-registration>)  [unwired: 2 in, 1 out]
  n16 = property class="XYGraph (strict)"(reference=w20, "Cursor.Cursor X"=w19, "Cursor.Cursor Y"=w19) -> (reference out=w18:refnum<vi>)  [unwired: 1 in, 1 out]
  n17 = control-ref of="cursor bracket: All, data window"() -> (w31:refnum<vi>)
  n18 = call "cursor window logic V2.vi"("cursor window action"=cursor_window_action."init", "cursor window in"=w31, "cursor window init"=w32) -> ("cursor window out"=w23:refnum<vi>)  [unwired: 7 in, 1 out]
  n19 = call "cursor window logic V2.vi"("cursor window action"=cursor_window_action."check", "cursor window in"=w23) -> ("cursor window out"=w21:refnum<vi>)  [unwired: 8 in, 1 out]
  n20 = while {
    tunnel: w44 -> [w53]
    tunnel: w26 -> [w51]
    tunnel: w21 -> [w47]
    tunnel: w18 -> [_]
    tunnel: w11 -> [w46]
    i -> [w48]
    stop <- FALSE stop-if-true
    n21 = Equal To 0?(x=w48) -> (x = 0?=w45:bool)
    n22 = event shown="[0] <calculate>: User Event" {
      selector: w53 -> [_ _]
      dyn-events: _ -> [_ _]
      timeout: 1 -> [_ _]
      tunnel: w51 -> [w67 _]
      tunnel: w47 -> [_ _]
      tunnel: w46 -> [w62 _]
      tunnel: w45 -> [w61 _]
      event User Event {
        # "all z"
        # "all omega"
        n23 = event-data() -> ("calculate"=w68:string)  [unwired: 1 in]
        n24 = local read "current resonance #"() -> (w54:i32)
        n25 = local read "pm lorentzian"() -> (w55:T5)
        n26 = control-ref of="Plot: All"() -> (w65:refnum<vi>)
        n27 = control-ref of="cursor bracket: All, data window"() -> (w56:refnum<vi>)
        n28 = for {
          N: 1 -> [_]
          tunnel: w68 -> [w86]
          tunnel: w67 -> [w85]
          shift-right: [w82] -> _
          shift-left: _ -> [w84]
          shift-right: [w81] -> _
          shift-left: _ -> [w83]
          tunnel: w56 -> [w80]
          tunnel: w65 -> [w79]
          tunnel: "Sweep folder path" -> [w78]
          tunnel: "Temperature (K)" -> [w77]
          tunnel: w54 -> [w76]
          tunnel: w62 -> [w75]
          tunnel: w61 -> [w74]
          tunnel: "parameters: complex fit" -> [w73]
          tunnel: "file path" -> [w72]
          tunnel: "scan monitor control" -> [w71]
          tunnel: "Magn Field (T)" -> [w70]
          tunnel: w55 -> [w69]
          n29 = case shown="\"scan for existing peaks\"" w86 {
            tunnel: w85 -> [_ _ _ _ _ _ _ _ _ _ _ w303 w321 w336 w350 _ _]
            tunnel: w84 -> [w93 w148 w196 w215 w234 w239 w251 w267 w278 w287 w289 w302 w320 w335 w349 w363 w372]
            tunnel: w83 -> [w92 w147 w195 w214 w233 w238 w250 w266 w277 w286 w288 w301 w319 w334 w348 w362 w371]
            tunnel: [w97 w148 w196 w215 w234 w239 w251 w267 w278 w287 w289 w302 w320 w335 w349 w363 w372] -> w82
            tunnel: [w96 w147 w195 w214 w233 w238 w250 w266 w277 w286 w288 w301 w319 w334 w348 w362 w371] -> w81
            tunnel: w80 -> [_ w146 _ _ w235 _ _ _ _ _ _ w304 w322 w337 w351 _ _]
            tunnel: w79 -> [_ _ _ _ _ _ _ _ _ _ _ _ _ _ _ _ _]
            tunnel: w78 -> [w95 w116 w192 w211 _ _ _ _ _ _ _ _ _ _ _ w356 w391]
            tunnel: w77 -> [_ w115 w188 w207 _ _ _ _ _ _ _ _ _ _ _ w354 _]
            tunnel: w76 -> [_ _ _ _ _ w237 w248 w260 w269 w280 _ w300 w318 w333 w339 _ _]
            tunnel: w75 -> [_ w145 _ _ w228 _ _ _ _ _ _ _ _ _ _ _ _]
            tunnel: w74 -> [_ w137 _ _ _ _ _ _ _ _ _ _ _ _ _ _ _]
            tunnel: w73 -> [_ w144 _ _ w227 _ _ _ _ _ _ _ _ _ _ _ _]
            tunnel: w72 -> [w89 _ _ _ _ _ _ _ _ _ _ _ _ _ _ _ _]
            tunnel: w71 -> [_ w113 _ _ _ _ _ _ _ _ _ _ _ _ _ _ _]
            tunnel: w70 -> [_ w112 _ _ _ _ _ _ _ _ _ _ _ _ _ _ _]
            tunnel: w69 -> [_ _ _ _ _ _ w249 w265 w276 w285 _ _ _ _ _ _ _]
            frame "calc:new file" {
              n30 = call "latest scan file.vi"("source"="source", "file path in"=w89, "sweep folder"=w95) -> ("temperature (K)"=w91:dbl, "file or folder exists?"=w94:bool, "file path out"=w90:path, "Magn Field (T)"=w87:dbl)  [unwired: 5 in]
              "scan file found" <- w94
              n31 = case shown="True" w94 {
                tunnel: [w99 w110] -> w97
                tunnel: [w98 w109] -> w96
                tunnel: w90 -> [_ w108]
                tunnel: w93 -> [w99 _]
                tunnel: w92 -> [w98 _]
                frame False {
                }
                frame True {
                  (unwired) TRUE ("read freq in")
                  (unwired) TRUE ("phase is normalized")
                  (unwired) 3 ("# columns in bin file")
                  (unwired) TRUE ("create bin file from dat")
                  # "Hz/kHz"
                  n32 = call "rus fit - load data file.vi"("file path"=w108, "read scan file"=T19 {"# columns"=3, "create bin file"=TRUE, "do not filter"=TRUE, "normalize phase"=TRUE, "read freq units"=enum."kHz"}) -> ("all:max omega"=→"all:max omega":dbl, "all:min omega"=→"all:min omega":dbl, "omega"=w110:dbl[], "x + iy"=w109:cdb[])  [unwired: 5 in, 1 out]
                  n33 = Complex To Re/Im(x + iy=w109) -> (x=w102:dbl[], y=w101:dbl[])
                  n34 = Bundle("omega"=w110, w102) -> (w103:cluster{"omega":dbl[], dbl[]})  [unwired: 1 in]
                  n35 = Bundle("omega"=w110, w101) -> (w104:cluster{"omega":dbl[], dbl[]})  [unwired: 1 in]
                  n36 = Build Array(w103, w104) -> (→"Plot: All":cluster{"omega":dbl[], dbl[]}[])
                }
              }
              n37 = local write "file path"(w90) -> ()
              n38 = local write "Magn Field (T)"(w87) -> ()
              n39 = local write "Temperature (K)"(w91) -> ()
            }
            frame "scan for existing peaks" {
              (unwired) 0 ("length")
              (unwired) 1.0 ("element")
              n40 = local read "Array of states"() -> (w143:T3[])
              n41 = local read "monitor state"() -> (w125:T2)
              n42 = Unbundle By Name(w113) -> ("iterate #"=w138:i32)
              n43 = call "monitor scan logic.vi"("Array"=w143, "monitor action"=monitor_action."read", "monitor state"=w125, "scan monitor control"=w113, "Sweep folder path"=w116, "temperature"=w115) -> ("Array out"=w128:T3[], "new freq"=w126:dbl[], "new gamma"=w127:dbl[], "monitor state OUT"=w133:T2)  [unwired: 6 in]
              n44 = call "monitor scan logic.vi"("Array"=w128, "monitor action"=monitor_action."global", "new freq IN"=w126, "new gamma IN"=w127, "monitor state"=w133, "scan monitor control"=w113) -> ("Array out"=w136:T3[], "new freq"=w135:dbl[], "new gamma"=w134:dbl[], "monitor state OUT"=w132:T2)  [unwired: 6 in]
              n45 = for {
                N: w138 -> [_]
                tunnel: w148 -> [w164]
                tunnel: w147 -> [w163]
                tunnel: w146 -> [w162]
                tunnel: w145 -> [w157]
                tunnel: w144 -> [w156]
                tunnel: w113 -> [w155]
                shift-right: [w153] -> w141
                shift-left: w135 -> [w160]
                shift-right: [w159] -> w140
                shift-left: w134 -> [w154]
                shift-right: [w158] -> w139
                shift-left: w136 -> [w151]
                shift-right: [w150] -> w131
                shift-left: w132 -> [w150]
                tunnel: "plot staff" -> [w149]
                n46 = for {
                  tunnel: w160 -> [w181] mode=indexing
                  tunnel: w162 -> [w184]
                  tunnel: w164 -> [w176]
                  tunnel: w163 -> [w175]
                  tunnel: [w182] -> w161 mode=indexing
                  tunnel: w154 -> [w178] mode=indexing
                  tunnel: w157 -> [w173]
                  tunnel: w156 -> [w172]
                  tunnel: w151 -> [w168] mode=indexing
                  tunnel: w149 -> [w166]
                  n47 = Unbundle By Name(w168) -> ("gamma-factor"=w167:dbl)
                  n48 = Multiply(x=w167, y=w178) -> (x*y=w180:dbl)
                  n49 = call "cursor window logic V2.vi"("cursor window action"=cursor_window_action."change cen&win", "window"=w180, "center"=w181, "cursor window in"=w184) -> ("cursor window out"=w169:T11)  [unwired: 6 in, 1 out]
                  n50 = call "peak -- find -- pm - V1.vi"("omega in"=w176, "z in"=w175, "cursor window"=w169, "parameters: complex fit"=w172, "plots: filter related"=w173, "plot staff ?"=w166) -> ("# points in window"=→"# of points in window":dbl, "good lorentzian"=w170:T5, "pm lorentzian"=w177:T5, "cp lorentzian"=w171:T5)  [unwired: 10 in]
                  n51 = Unbundle By Name(w170) -> ("omega(0)"=w174:dbl, "Gamma"=w179:dbl)
                  n52 = local write "pm lorentzian"(w177) -> ()
                  n53 = local write "cp lorentzian"(w171) -> ()
                  n54 = Bundle By Name(cluster=w168, "exp"=w181, "found"=w174, "gamma"=w178, "gamma found"=w179) -> (w182:T3)
                }
                n55 = call "monitor scan logic.vi"("Array"=w161, "monitor action"=monitor_action."monitor", "scan monitor control"=w155) -> ("Array out"=w158:T3[], "new freq"=w153:dbl[], "new gamma"=w159:dbl[])  [unwired: 9 in, 1 out]
              }
              n56 = local write "OLD gamma"(w127) -> ()
              n57 = local write "OLD freq"(w126) -> ()
              n58 = call "monitor scan logic.vi"("Array"=w139, "monitor action"=monitor_action."interpolate", "init"=w137, "new freq IN"=w141, "new gamma IN"=w140, "monitor state"=w131, "scan monitor control"=w113) -> ("Array out"=w124:T3[], "new freq"=w122:dbl[], "new gamma"=w121:dbl[], "monitor state OUT"=w120:T2)  [unwired: 5 in]
              n59 = call "monitor scan logic.vi"("Array"=w124, "monitor action"=monitor_action."overwrite", "new freq IN"=w122, "Magn Field (T)"=w112, "new gamma IN"=w121, "monitor state"=w120, "scan monitor control"=w113, "Sweep folder path"=w116, "temperature"=w115) -> ("Array out"=w123:T3[], "new freq"=w117:dbl[], "new gamma"=w118:dbl[], "monitor state OUT"=w119:T2)  [unwired: 3 in]
              n60 = local write "Array of states"(w123) -> ()
              n61 = local write "NEW freq"(w117) -> ()
              n62 = local write "NEW gamma"(w118) -> ()
              n63 = local write "monitor state"(w119) -> ()
            }
            frame "dump OLD peak gamma" {
              w191 = enum16{"append", "overwrite"}."overwrite" ("append/overwrite")
              n64 = local read "OLD gamma"() -> (w189:dbl[])
              n65 = local read "OLD freq"() -> (w193:dbl[])
              n66 = case shown="\"WORK\"" "overwrite (d)" {
                tunnel: [ctl_--_name_dispatcher_--_action."peak frequency DUMP" ("ctl name dispatch") ctl_--_name_dispatcher_--_action."peak frequency" ("ctl name dispatch")] -> w194
                tunnel: [ctl_--_name_dispatcher_--_action."peak gamma DUMP" ("ctl name dispatch") ctl_--_name_dispatcher_--_action."peak gamma" ("ctl name dispatch")] -> w190
                tunnel: [enum16{"DUMP", "WORK", ""}."DUMP" ("dump/work") enum16{"DUMP", "WORK", ""}."DUMP" ("dump/work")] -> w186
                tunnel: [FALSE ("overwriting !!") FALSE ("overwriting !!")] -> w185
                frame "DUMP", Default {
                }
                frame "WORK" {
                }
              }
              n67 = call "PID append overwrite.vi"("temperature"=w188, "append/overwrite"=w191, "PID freq"=w193, "ctl kind IN"=w194, "sweep folder"=w192) -> ()  [unwired: 6 in, 1 out]
              n68 = call "PID append overwrite.vi"("temperature"=w188, "append/overwrite"=w191, "PID freq"=w189, "ctl kind IN"=w190, "sweep folder"=w192) -> ()  [unwired: 6 in, 1 out]
              n69 = local write "overwriting !!"(w185) -> ()
              n70 = local write "overwrite (d)"(w186) -> ()
            }
            frame "dump NEW peak gamma" {
              w210 = enum16{"append", "overwrite"}."overwrite" ("append/overwrite")
              n71 = local read "NEW gamma"() -> (w208:dbl[])
              n72 = local read "NEW freq"() -> (w212:dbl[])
              n73 = case shown="\"DUMP\", Default" "dump/work NEW (\"n\")" {
                tunnel: [ctl_--_name_dispatcher_--_action."peak frequency DUMP" ("ctl name dispatch") ctl_--_name_dispatcher_--_action."peak frequency" ("ctl name dispatch")] -> w213
                tunnel: [ctl_--_name_dispatcher_--_action."peak gamma DUMP" ("ctl name dispatch") ctl_--_name_dispatcher_--_action."peak gamma" ("ctl name dispatch")] -> w209
                tunnel: [enum16{"DUMP", "WORK", ""}."DUMP" ("dump/work") enum16{"DUMP", "WORK", ""}."DUMP" ("dump/work")] -> w205
                frame "DUMP", Default {
                }
                frame "WORK" {
                }
              }
              n74 = call "PID append overwrite.vi"("temperature"=w207, "append/overwrite"=w210, "PID freq"=w212, "ctl kind IN"=w213, "sweep folder"=w211) -> ()  [unwired: 6 in, 1 out]
              n75 = call "PID append overwrite.vi"("temperature"=w207, "append/overwrite"=w210, "PID freq"=w208, "ctl kind IN"=w209, "sweep folder"=w211) -> ()  [unwired: 6 in, 1 out]
              n76 = local write "dump/work NEW (\"n\")"(w205) -> ()
            }
            frame "one peak" {
              n77 = call "cursor window logic V2.vi"("cursor window action"=cursor_window_action."check", "cursor window in"=w235) -> ("cursor window out"=w232:T11)  [unwired: 8 in, 1 out]
              n78 = Unbundle By Name(w232) -> ("center"=→"window center (kHz)":dbl, "window"=→"window width (kHz)":dbl)
              n79 = call "peak -- find -- pm - V1.vi"("omega in"=w234, "z in"=w233, "cursor window"=w232, "parameters: complex fit"=w227, "plots: filter related"=w228, "plot staff ?"=enum16{"plot", "do not plot", "a"}."plot", "just guess?"="use fast fit?") -> ("# points in window"=w225:dbl, "good lorentzian"=→"good lorentzian":T5, "pm lorentzian"=w229:T5, "cp lorentzian"=w226:T5)  [unwired: 9 in]
              n80 = local write "# of points in window"(w225) -> ()
              n81 = local write "pm lorentzian"(w229) -> ()
              n82 = local write "cp lorentzian"(w226) -> ()
            }
            frame "save search window" {
              n83 = local read "OLD gamma"() -> (w242:dbl[])
              n84 = local read "OLD freq"() -> (w243:dbl[])
              n85 = in-place {
                n86 = in-place-array #1(w243, w237) -> ()  [unwired: 1 out]
                n87 = local read "window center (kHz)"() -> (w245:dbl)
                n88 = in-place-array #1(w245) -> (w240:dbl[])  [unwired: 1 out]
              }
              n89 = in-place {
                n90 = in-place-array #2(w242, w237) -> ()  [unwired: 1 out]
                n91 = local read "window width (kHz)"() -> (w244:dbl)
                n92 = in-place-array #2(w244) -> (w241:dbl[])  [unwired: 1 out]
              }
              n93 = local write "OLD freq"(w240) -> ()
              n94 = local write "OLD gamma"(w241) -> ()
            }
            frame "save current lorentzian" {
              n95 = local read "OLD gamma"() -> (w254:dbl[])
              n96 = local read "OLD freq"() -> (w255:dbl[])
              n97 = Unbundle By Name(w249) -> ("omega(0)"=w247:dbl, "Gamma"=w246:dbl)
              n98 = in-place {
                in-place-border: w247 -> [w257]
                n99 = in-place-array #3(w255, w248) -> ()  [unwired: 1 out]
                n100 = in-place-array #3(w257) -> (w252:dbl[])  [unwired: 1 out]
              }
              n101 = in-place {
                in-place-border: w246 -> [w256]
                n102 = in-place-array #4(w254, w248) -> ()  [unwired: 1 out]
                n103 = in-place-array #4(w256) -> (w253:dbl[])  [unwired: 1 out]
              }
              n104 = local write "OLD freq"(w252) -> ()
              n105 = local write "OLD gamma"(w253) -> ()
            }
            frame "insert resonance -- from lorentzian" {
              n106 = local read "OLD gamma"() -> (w262:dbl[])
              n107 = local read "OLD freq"() -> (w264:dbl[])
              n108 = Unbundle By Name(w265) -> ("omega(0)"=w259:dbl, "Gamma"=w258:dbl)
              n109 = Insert Into Array(array=w264, index=w260, new element=w259) -> (w263:dbl[])
              n110 = Insert Into Array(array=w262, index=w260, new element=w258) -> (w261:dbl[])
              n111 = local write "OLD freq"(w263) -> ()
              n112 = local write "OLD gamma"(w261) -> ()
            }
            frame "insert resonance -- from window" {
              n113 = local read "window center (kHz)"() -> (w274:dbl)
              n114 = local read "window width (kHz)"() -> (w270:dbl)
              n115 = local read "OLD gamma"() -> (w272:dbl[])
              n116 = local read "OLD freq"() -> (w275:dbl[])
              n117 = Unbundle By Name(w276) -> ()  [unwired: 2 out]
              n118 = call "array -- incert after.vi"("index"=w269, "Array"=w275, "number"=w274) -> ("array out"=w273:dbl[])  [unwired: 7 in, 1 out]
              n119 = call "array -- incert after.vi"("index"=w269, "Array"=w272, "number"=w270) -> ("array out"=w271:dbl[], "new index"=w268:i32)  [unwired: 7 in]
              n120 = local write "OLD freq"(w273) -> ()
              n121 = local write "OLD gamma"(w271) -> ()
              n122 = local write "current resonance #"(w268) -> ()
            }
            frame "delete resonance" {
              w279 = 1 ("length")
              n123 = local read "OLD gamma"() -> (w282:dbl[])
              n124 = local read "OLD freq"() -> (w284:dbl[])
              n125 = Unbundle By Name(w285) -> ()  [unwired: 2 out]
              n126 = Delete From Array(array=w284, length=w279, index=w280) -> (array with subset deleted=w283:dbl[])  [unwired: 1 out]
              n127 = Delete From Array(array=w282, length=w279, index=w280) -> (array with subset deleted=w281:dbl[])  [unwired: 1 out]
              n128 = local write "OLD freq"(w283) -> ()
              n129 = local write "OLD gamma"(w281) -> ()
            }
            frame "aaa", Default {
            }
            frame "jump to a PID peak" {
              w291 = "one peak"  # event data
              n130 = local read "OLD freq"() -> (w305:dbl[])
              n131 = case shown="True" TRUE {
                tunnel: w300 -> [w306 w308]
                tunnel: [w306 w307] -> w299
                frame False {
                }
                frame True {
                  n132 = Increment(x=w308) -> (x+1=w307:i32)
                }
              }
              n133 = Generate User Event(user event=w303, event data cluster=w291) -> ()  [unwired: 2 in, 2 out]
              n134 = Array Size(array=w305) -> (size(s)=w296:i32)
              n135 = Equal To 0?(x=w296) -> (x = 0?=w298:bool)
              n136 = Select(t=1, s=w298, f=w296) -> (s? t:f=w295:i32)
              n137 = Quotient & Remainder(x=w299, y=w295) -> (x-y*floor(x/y)=w292:i32)  [unwired: 1 out]
              n138 = local write "current resonance #"(w292) -> ()
              n139 = Index Array(array=w305, index=w292) -> (element=w293:dbl)
              n140 = call "cursor window logic V2.vi"("cursor window action"=cursor_window_action."change center", "center"=w293, "cursor window in"=w304) -> ()  [unwired: 7 in, 2 out]
            }
            frame "next resonance" {
              (unwired) TRUE
              w309 = "one peak"  # event data
              n141 = local read "OLD freq"() -> (w323:dbl[])
              n142 = Generate User Event(user event=w321, event data cluster=w309) -> ()  [unwired: 2 in, 2 out]
              n143 = Increment(x=w318) -> (x+1=w317:i32)
              n144 = Array Size(array=w323) -> (size(s)=w314:i32)
              n145 = Equal To 0?(x=w314) -> (x = 0?=w316:bool)
              n146 = Select(t=1, s=w316, f=w314) -> (s? t:f=w313:i32)
              n147 = Quotient & Remainder(x=w317, y=w313) -> (x-y*floor(x/y)=w310:i32)  [unwired: 1 out]
              n148 = local write "current resonance #"(w310) -> ()
              n149 = Index Array(array=w323, index=w310) -> (element=w311:dbl)
              n150 = call "cursor window logic V2.vi"("cursor window action"=cursor_window_action."change center", "center"=w311, "cursor window in"=w322) -> ()  [unwired: 7 in, 2 out]
            }
            frame "prev resonance" {
              (unwired) TRUE
              w324 = "one peak"  # event data
              n151 = local read "OLD freq"() -> (w338:dbl[])
              n152 = Generate User Event(user event=w336, event data cluster=w324) -> ()  [unwired: 2 in, 2 out]
              n153 = Decrement(x=w333) -> (x-1=w332:i32)
              n154 = Array Size(array=w338) -> (size(s)=w329:i32)
              n155 = Equal To 0?(x=w329) -> (x = 0?=w331:bool)
              n156 = Select(t=1, s=w331, f=w329) -> (s? t:f=w328:i32)
              n157 = Quotient & Remainder(x=w332, y=w328) -> (x-y*floor(x/y)=w325:i32)  [unwired: 1 out]
              n158 = local write "current resonance #"(w325) -> ()
              n159 = Index Array(array=w338, index=w325) -> (element=w326:dbl)
              n160 = call "cursor window logic V2.vi"("cursor window action"=cursor_window_action."change center", "center"=w326, "cursor window in"=w337) -> ()  [unwired: 7 in, 2 out]
            }
            frame "jump to a resonance" {
              (unwired) TRUE
              w340 = "one peak"  # event data
              n161 = local read "OLD freq"() -> (w352:dbl[])
              n162 = Generate User Event(user event=w350, event data cluster=w340) -> ()  [unwired: 2 in, 2 out]
              n163 = Array Size(array=w352) -> (size(s)=w345:i32)
              n164 = Equal To 0?(x=w345) -> (x = 0?=w347:bool)
              n165 = Select(t=1, s=w347, f=w345) -> (s? t:f=w344:i32)
              n166 = Quotient & Remainder(x=w339, y=w344) -> (x-y*floor(x/y)=w341:i32)  [unwired: 1 out]
              n167 = local write "current resonance #"(w341) -> ()
              n168 = Index Array(array=w352, index=w341) -> (element=w342:dbl)
              n169 = call "cursor window logic V2.vi"("cursor window action"=cursor_window_action."change center", "center"=w342, "cursor window in"=w351) -> ()  [unwired: 7 in, 2 out]
            }
            frame "reread resonances" {
              (unwired) TRUE
              n170 = call "PID -- read interpolate.vi"("sweep folder path"=w356, "ctl PID file IN"=ctl_--_name_dispatcher_--_action."peak frequency" ("ctl name dispatch"), "temperature"=w354) -> ("sweep folder path out"=w360:path, "PID freq"=w355:dbl[], "length out"=w357:i32)  [unwired: 11 in, 3 out]
              n171 = call "PID -- read interpolate.vi"("sweep folder path"=w360, "ctl PID file IN"=ctl_--_name_dispatcher_--_action."peak gamma" ("ctl name dispatch"), "length"=w357, "default"=1.0 ("element")) -> ("PID freq"=w353:dbl[])  [unwired: 10 in, 5 out]
              n172 = local write "OLD gamma"(w353) -> ()
              n173 = local write "OLD freq"(w355) -> ()
            }
            frame "append a line" {
              (unwired) "ctl_PID_peak_gamma_NEW.dat" ("freq PID file IN")
              w393 = 0.0 ("lower")
              n174 = call "ctl -- name dispatcher.vi"("ctl name dispatch"=ctl_--_name_dispatcher_--_action."peak frequency TEST") -> ("ctl file name"=w368:string)  [unwired: 8 in, 2 out]
              n175 = call "ctl -- name dispatcher.vi"("ctl name dispatch"=ctl_--_name_dispatcher_--_action."peak gamma TEST") -> ("ctl file name"=w366:string)  [unwired: 8 in, 2 out]
              n176 = local read "pm lorentzian"() -> (w396:T5)
              n177 = call "ctl -- name dispatcher.vi"("ctl name dispatch"=ctl_--_name_dispatcher_--_action."peak freq gamma TEST") -> ("ctl file name"=w364:string)  [unwired: 8 in, 2 out]
              n178 = call "file -- 9w path.vi"("sweep folder"=w391) -> ("9w path"=w380:path)  [unwired: 10 in]
              n179 = Unbundle By Name(w396) -> ("omega(0)"=w395:dbl, "Gamma"=w394:dbl)
              n180 = Build Path(base path=w380, name or relative path=w364) -> (appended path=w370:path)
              n181 = Build Path(base path=w380, name or relative path=w366) -> (appended path=w382:path)
              n182 = Build Path(base path=w380, name or relative path=w368) -> (appended path=w390:path)
              n183 = call "Q -- check range -- i -- real.vi"("lower"=w393, "default"=1.0, "number"=w394) -> ("number in range"=w381:dbl)  [unwired: 6 in, 2 out]
              n184 = call "Q -- check range -- i -- real.vi"("lower"=w393, "default"=w393, "number"=w395) -> ("number in range"=w388:dbl)  [unwired: 6 in, 2 out]
              n185 = Number To Fractional String(number=w381) -> (F-format string=w375:string)  [unwired: 3 in]
              n186 = Number To Fractional String(number=w388) -> (F-format string=w376:string)  [unwired: 3 in]
              n187 = Build Array(w375) -> (w384:string[])
              n188 = Build Array(w376) -> (w387:string[])
              n189 = call-poly <vilib>:"Write To Spreadsheet File.vi"("delimiter (\\t)"="\r", "append to file? (new file:F)"=TRUE, "1D data"=w384, "file path (dialog if empty)"=w382) -> ()  [unwired: 4 in, 1 out]
              n190 = call-poly <vilib>:"Write To Spreadsheet File.vi"("delimiter (\\t)"="\r", "append to file? (new file:F)"=TRUE, "1D data"=w387, "file path (dialog if empty)"=w390) -> ()  [unwired: 4 in, 1 out]
              n191 = Concatenate Strings(w376, "\t", w375) -> (w374:string)
              n192 = Build Array(w374) -> (w378:string[])
              n193 = call-poly <vilib>:"Write To Spreadsheet File.vi"("delimiter (\\t)"="\r", "append to file? (new file:F)"=TRUE, "1D data"=w378, "file path (dialog if empty)"=w370) -> ()  [unwired: 4 in, 1 out]
            }
          }
        }
      }
      event Timeout {
        n194 = event-data() -> ()  [unwired: 1 in, 2 out]
      }
    }
    n195 = Wait (ms)(milliseconds to wait=u32 111) -> ()  [unwired: 1 out]
  }
  n196 = Create User Event(user event datatype=w28) -> (user event=w27:refnum<user-event>)  [unwired: 1 in, 1 out]
  n197 = register-events(w27) -> (reference out=w29:refnum<event-registration>)  [unwired: 2 in, 1 out]
  n198 = control-ref of="timer \"o\""() -> (w25:refnum<vi>)
  n199 = while {
    tunnel: w29 -> [w404]
    tunnel: w26 -> [w403]
    stop <- FALSE stop-if-true
    n200 = local read "good lorentzian"() -> (w397:T5)
    n201 = local read "cp lorentzian"() -> (w400:T5)
    n202 = control-ref of="Plot: complex plane"() -> (w399:refnum<vi>)
    n203 = control-ref of="cursor bracket: All, data window"() -> (w398:refnum<vi>)
    n204 = event shown="[1] Key Down" {
      selector: w404 -> [_ _ _ _ _ _ _ _]
      dyn-events: _ -> [_ _ _ _ _ _ _ _]
      timeout: _ -> [_ _ _ _ _ _ _ _]
      tunnel: w403 -> [_ w411 _ _ _ w503 _ _]
      tunnel: w398 -> [_ w410 _ _ w501 _ _ _]
      tunnel: w400 -> [_ w406 _ _ _ _ _ w521]
      tunnel: w399 -> [_ w405 _ _ _ _ _ w519]
      tunnel: w397 -> [_ _ _ _ _ _ w508 _]
      event Timeout {
        n205 = event-data() -> ()  [unwired: 1 in, 2 out]
      }
      event Key Down {
        n206 = event-data() -> ("Char"=w408:i16, "VKey"=w412:T12)  [unwired: 1 in]
        "Char" <- w408
        "VKey" <- w412
        n207 = Build Array(w408) -> (w409:i16[])
        n208 = Byte Array To String(unsigned byte array=w409) -> (string=w407:string)
        n209 = case shown="\"ASCII\", Default" w412 {
          selector: w412 -> [_ _ _ _ w479]
          tunnel: w408 -> [_ _ _ _ _]
          tunnel: w411 -> [w417 _ w473 w475 w478]
          tunnel: w410 -> [w416 _ _ _ w480]
          tunnel: w407 -> [w415 _ _ _ _]
          tunnel: w406 -> [w414 _ _ _ _]
          tunnel: w405 -> [w413 _ _ _ _]
          frame "ASCII", Default {
            n210 = case shown="\"U\"" w415 {
              tunnel: w417 -> [_ _ _ w428 w430 _ _ w436 _ w442 w444 w446 _ w459 w461 w463 w467 w470]
              tunnel: w416 -> [_ _ w425 _ _ w431 w433 _ _ _ _ _ _ _ _ _ _ _]
              tunnel: w414 -> [_ _ _ _ _ _ _ _ _ _ _ _ w447 _ _ _ _ _]
              tunnel: w413 -> [_ _ _ _ _ _ _ _ _ _ _ _ w448 _ _ _ _ _]
              frame "0", Default {
              }
              frame "*" {
                # "*"
                n211 = local read "overwrite (d)"() -> (w420:enum16{"DUMP", "WORK", ""})
                n212 = case shown="\"DUMP\", Default" w420 {
                  tunnel: [enum16{"DUMP", "WORK", ""}."WORK" ("overwrite dump/work (\"d\")") enum16{"DUMP", "WORK", ""}."DUMP" ("overwrite dump/work (\"d\")")] -> w419
                  tunnel: [TRUE ("overwriting !!") FALSE ("overwriting !!")] -> w418
                  frame "DUMP", Default {
                  }
                  frame "WORK" {
                  }
                }
                n213 = local write "overwrite (d)"(w419) -> ()
                n214 = local write "overwriting !!"(w418) -> ()
              }
              frame "?" {
                # "?"
                n215 = call "cursor window logic V2.vi"("cursor window action"=cursor_window_action."zoom X", "cursor window in"=w425) -> ()  [unwired: 8 in, 2 out]
              }
              frame "o" {
                # "o"
                n216 = Generate User Event(user event=w428, event data cluster="calc:new file" ("event data")) -> ()  [unwired: 2 in, 2 out]
              }
              frame "\\" {
                # "\\"
                n217 = Generate User Event(user event=w430, event data cluster="jump to a PID peak" ("event data")) -> ()  [unwired: 2 in, 2 out]
              }
              frame "a" {
                # "\"a\" - zoom out"
                n218 = call "cursor window logic V2.vi"("cursor window action"=cursor_window_action."zoom to all data", "cursor window in"=w431) -> ()  [unwired: 8 in, 2 out]
              }
              frame "c" {
                # "\"c\"- for cursor"
                n219 = call "cursor window logic V2.vi"("cursor window action"=cursor_window_action."check", "cursor window in"=w433) -> ()  [unwired: 8 in, 2 out]
              }
              frame "d" {
                # "d"
                n220 = Generate User Event(user event=w436, event data cluster="dump OLD peak gamma" ("event data")) -> ()  [unwired: 2 in, 2 out]
              }
              frame "e" {
                # "e"
                n221 = local read "Tab : monitor"() -> (w438:enum32{"main", "EDIT"})
                n222 = case shown="\"main\", Default" w438 {
                  tunnel: [enum32{"main", "EDIT"}."EDIT" ("Tab : monitor") enum32{"main", "EDIT"}."main" ("Tab : monitor")] -> w437
                  frame "main", Default {
                  }
                  frame "EDIT" {
                  }
                }
                n223 = local write "Tab : monitor"(w437) -> ()
              }
              frame "n" {
                # "n"
                n224 = Generate User Event(user event=w442, event data cluster="dump NEW peak gamma" ("event data")) -> ()  [unwired: 2 in, 2 out]
              }
              frame "q" {
                # "n"
                n225 = Generate User Event(user event=w444, event data cluster="save search window" ("event data")) -> ()  [unwired: 2 in, 2 out]
              }
              frame "Q" {
                n226 = Generate User Event(user event=w446, event data cluster="save current lorentzian" ("event data")) -> ()  [unwired: 2 in, 2 out]
              }
              frame " " {
                n227 = Unbundle By Name(w447) -> ("4corners.z center"=w456:cdb)
                n228 = local read "scale gauge: Plot: complex plane"() -> (w457:dbl)
                n229 = Complex To Re/Im(x + iy=w456) -> (x=w455:dbl, y=w454:dbl)
                n230 = Negate(x=w457) -> (-x=w449:dbl)
                n231 = Add(x=w454, y=w449) -> (x+y=w453:dbl)
                n232 = Add(x=w455, y=w457) -> (x+y=w451:dbl)
                n233 = Add(x=w455, y=w449) -> (x+y=w450:dbl)
                n234 = Add(x=w454, y=w457) -> (x+y=w452:dbl)
                n235 = property on="Property Node" class="XYGraph (strict)"(reference=w448, "XScale.Minimum"=w450, "XScale.Maximum"=w451, "YScale.Maximum"=w452, "YScale.Minimum"=w453) -> ()  [unwired: 1 in, 2 out]
              }
              frame "y" {
                # "y"
                n236 = Generate User Event(user event=w459, event data cluster="append a line" ("event data")) -> ()  [unwired: 2 in, 2 out]
              }
              frame "I" {
                # "y"
                n237 = Generate User Event(user event=w461, event data cluster="insert resonance -- from window" ("event data")) -> ()  [unwired: 2 in, 2 out]
              }
              frame "R" {
                # "y"
                n238 = Generate User Event(user event=w463, event data cluster="delete resonance" ("event data")) -> ()  [unwired: 2 in, 2 out]
              }
              frame "U" {
                n239 = for {
                  N: 100 -> [_]
                  tunnel: [w468] -> w464 mode=indexing
                  i -> [w468]
                }
                "index" <- w464
                "index -- main" <- w464
                n240 = Generate User Event(user event=w467, event data cluster="reread resonances" ("event data")) -> ()  [unwired: 2 in, 2 out]
              }
              frame "v" {
                # "v"
                n241 = Generate User Event(user event=w470, event data cluster="scan for existing peaks" ("event data")) -> ()  [unwired: 2 in, 2 out]
              }
            }
          }
          frame "Escape" {
            n242 = local read "use fast fit?"() -> (w471:bool)
            n243 = Not(x=w471) -> (.not. x?=w472:bool)
            n244 = local write "use fast fit?"(w472) -> ()
          }
          frame "PageUp" {
            n245 = Generate User Event(user event=w473, event data cluster="next resonance" ("event data")) -> ()  [unwired: 2 in, 2 out]
          }
          frame "PageDown" {
            n246 = Generate User Event(user event=w475, event data cluster="prev resonance" ("event data")) -> ()  [unwired: 2 in, 2 out]
          }
          frame "Up".."Right" {
            n247 = case shown="\"Left\"" w479 {
              tunnel: w480 -> [w481 w483 w485 w488]
              frame "Right", Default {
                n248 = call "cursor window logic V2.vi"("cursor window action"=cursor_window_action."move right", "cursor window in"=w481) -> ()  [unwired: 8 in, 2 out]
              }
              frame "Left" {
                n249 = call "cursor window logic V2.vi"("cursor window action"=cursor_window_action."move left", "cursor window in"=w483) -> ()  [unwired: 8 in, 2 out]
              }
              frame "Up" {
                n250 = call "cursor window logic V2.vi"("cursor window action"=cursor_window_action."broaden", "cursor window in"=w485) -> ()  [unwired: 8 in, 2 out]
              }
              frame "Down" {
                n251 = call "cursor window logic V2.vi"("cursor window action"=cursor_window_action."shrink", "cursor window in"=w488) -> ()  [unwired: 8 in, 2 out]
              }
            }
            n252 = Generate User Event(user event=w478, event data cluster="one peak" ("event data")) -> ()  [unwired: 2 in, 2 out]
          }
        }
      }
      event "overwrite (d)": Value Change {
        n253 = event-data() -> ("NewVal"=w490:enum16{"DUMP", "WORK", ""})  [unwired: 1 in]
        n254 = case shown="\"DUMP\", Default" w490 {
          tunnel: [FALSE ("overwriting !!") TRUE ("overwriting !!")] -> w489
          frame "DUMP", Default {
          }
          frame "WORK" {
          }
        }
        n255 = local write "overwriting !!"(w489) -> ()
      }
      event "autopilot": Value Change {
        n256 = event-data() -> ("NewVal"=w495:enum32{"on", "off"})  [unwired: 1 in]
        n257 = local read "scan monitor control"() -> (w494:T1)
        n258 = case shown="\"on\"" w495 {
          tunnel: w494 -> [w498 w499]
          tunnel: [w496 w499] -> w493
          frame "on" {
            n259 = Bundle By Name(cluster=w498, "overwrite?"=TRUE) -> (w496:T1)
          }
          frame "off", Default {
          }
        }
        n260 = local write "scan monitor control"(w493) -> ()
      }
      event "Plot: All": Cursor Move {
        n261 = event-data() -> ("CursIdx"=w500:i32)  [unwired: 1 in, 3 out]
        n262 = call "cursor window logic V2.vi"("CursIdx"=w500, "cursor window action"=cursor_window_action."cursor moves", "cursor window in"=w501) -> ()  [unwired: 7 in, 2 out]
      }
      event "Plot: All": Cursor Release {
        n263 = event-data() -> ("CursIdx"=w504:i32)  [unwired: 1 in, 3 out]
        n264 = case shown="0..2" w504 {
          tunnel: w503 -> [_ w505]
          frame 3, Default {
          }
          frame 0..2 {
            w506 = "one peak"  # event data
            n265 = Generate User Event(user event=w505, event data cluster=w506) -> ()  [unwired: 2 in, 2 out]
          }
        }
      }
      event "scale gauge: Plot: complex plane - filter": Value Change {
        n266 = event-data() -> ("NewVal"=w510:dbl)  [unwired: 1 in]
        n267 = Unbundle By Name(w508) -> ("4corners.z center"=w509:cdb)
        n268 = Unbundle By Name(w508) -> ("4corners"=→"4corners":T6)
        n269 = Complex To Re/Im(x + iy=w509) -> (x=w512:dbl, y=w513:dbl)
        n270 = Negate(x=w510) -> (-x=w518:dbl)
        n271 = control-ref of="Plot: complex plane - filter"() -> (w511:refnum<vi>)
        n272 = Add(x=w513, y=w518) -> (x+y=w514:dbl)
        n273 = Add(x=w512, y=w510) -> (x+y=w516:dbl)
        n274 = Add(x=w512, y=w518) -> (x+y=w517:dbl)
        n275 = Add(x=w513, y=w510) -> (x+y=w515:dbl)
        n276 = property on="Property Node" class="XYGraph (strict)"(reference=w511, "XScale.Minimum"=w517, "XScale.Maximum"=w516, "YScale.Maximum"=w515, "YScale.Minimum"=w514) -> ()  [unwired: 1 in, 2 out]
      }
      event "scale gauge: Plot: complex plane": Value Change {
        n277 = event-data() -> ("NewVal"=w522:dbl)  [unwired: 1 in]
        n278 = Unbundle By Name(w521) -> ("4corners.z center"=w520:cdb)
        n279 = Complex To Re/Im(x + iy=w520) -> (x=w523:dbl, y=w524:dbl)
        n280 = Negate(x=w522) -> (-x=w529:dbl)
        n281 = Add(x=w524, y=w529) -> (x+y=w525:dbl)
        n282 = Add(x=w523, y=w522) -> (x+y=w527:dbl)
        n283 = Add(x=w523, y=w529) -> (x+y=w528:dbl)
        n284 = Add(x=w524, y=w522) -> (x+y=w526:dbl)
        n285 = property on="Property Node" class="XYGraph (strict)"(reference=w519, "XScale.Minimum"=w528, "XScale.Maximum"=w527, "YScale.Maximum"=w526, "YScale.Minimum"=w525) -> ()  [unwired: 1 in, 2 out]
      }
    }
    n286 = Wait (ms)(milliseconds to wait=u32 31) -> ()  [unwired: 1 out]
  }
  n287 = control-ref of="timer \"v\""() -> (w24:refnum<vi>)
  n288 = control-ref of="timer  \"update\""() -> (w7:refnum<vi>)
  n289 = call "slider timer .vi"("action"=w6, "timer ref"=w7) -> ("timer out"=w5:refnum<vi>)  [unwired: 7 in, 2 out]
  n290 = call "slider timer .vi"("action"=w6, "timer ref"=w25) -> ("timer out"=w42:refnum<vi>)  [unwired: 7 in, 2 out]
  n291 = call "slider timer .vi"("action"=w6, "timer ref"=w24) -> ("timer out"=w3:refnum<vi>)  [unwired: 7 in, 2 out]
  n292 = local read "file path"() -> (w4:path)
  n293 = call "slider timer .vi"("action"=countdown_control."stop", "timer ref"=w3) -> ("timer out"=w2:refnum<vi>)  [unwired: 7 in, 2 out]
  n294 = while {
    tunnel: w26 -> [w545]
    shift-right: [w551] -> _
    shift-left: w42 -> [w552]
    shift-right: [w549] -> _
    shift-left: w2 -> [w550]
    shift-right: [w543] -> _
    shift-left: w5 -> [w544]
    shift-right: [w540] -> _
    shift-left: w4 -> [w541]
    stop <- FALSE stop-if-true
    (unwired) 0
    w547 = countdown_control."check" ("action")
    n295 = case shown="\"watch\", Default" "\"o\" timer selector" {
      tunnel: [TRUE FALSE] -> w532
      frame "watch", Default {
      }
      frame "absol" {
      }
    }
    n296 = call "slider timer .vi"("action"=w547, "timer ref"=w552) -> ("tic"=w536:bool, "timer out"=w551:refnum<vi>)  [unwired: 7 in, 1 out]
    n297 = call "slider timer .vi"("action"=countdown_control."check", "timer ref"=w544) -> ("tic"=w539:bool, "timer out"=w543:refnum<vi>)  [unwired: 7 in, 1 out]
    n298 = case shown="\"on\"" "autopilot" {
      tunnel: [FALSE TRUE] -> w530
      frame "off", Default {
      }
      frame "on" {
      }
    }
    n299 = Compound Arithmetic op=AND(w539, w532, w530) -> (w538:bool)
    n300 = Wait (ms)(milliseconds to wait=u32 123) -> ()  [unwired: 1 out]
    n301 = case shown="True" w538 {
      tunnel: w541 -> [w564 w568]
      tunnel: [w564 w566] -> w540
      tunnel: [FALSE w565] -> w537
      frame False {
      }
      frame True {
        n302 = local read "Sweep folder path"() -> (w573:path)
        n303 = call "latest scan file.vi"("source"=enum16{"last scan file", "manual"}."last scan file", "file path in"=w568, "sweep folder"=w573) -> ("temperature (K)"=w572:dbl, "file or folder exists?"=w567:bool, "file path out"=w569:path)  [unwired: 5 in, 1 out]
        n304 = Not Equal?(x=w569, y=w568) -> (x != y?=w570:bool)
        n305 = And(x=w567, y=w570) -> (x .and. y?=w565:bool)
        n306 = local write "Temperature (K)"(w572) -> ()
        n307 = Select(t=w569, s=w565, f=w568) -> (s? t:f=w566:path)
        n308 = local write "file path"(w566) -> ()
        n309 = local write "scan file found"(w567) -> ()
      }
    }
    n310 = case shown="True" w532 {
      tunnel: [w561 w562] -> w535
      tunnel: w537 -> [_ w562]
      tunnel: w536 -> [w561 _]
      frame False {
      }
      frame True {
      }
    }
    n311 = Select(t=countdown_control."reset once" ("action"), s=w535, f=w547) -> (s? t:f=w546:T16)
    n312 = call "slider timer .vi"("action"=w546, "timer ref"=w550) -> ("tic"=w534:bool, "timer out"=w549:refnum<vi>)  [unwired: 7 in, 1 out]
    n313 = And(x=w530, y=w534) -> (x .and. y?=w553:bool)
    n314 = case shown="True" w553 {
      tunnel: w545 -> [_ w574]
      frame False {
      }
      frame True {
        w575 = "scan for existing peaks"  # calculate
        n315 = Generate User Event(user event=w574, event data cluster=w575) -> ()  [unwired: 2 in, 2 out]
      }
    }
    n316 = And(x=w530, y=w535) -> (x .and. y?=w554:bool)
    n317 = case shown="True" w554 {
      tunnel: w545 -> [_ w577]
      frame False {
      }
      frame True {
        w576 = "calc:new file"  # calculate
        n318 = Generate User Event(user event=w577, event data cluster=w576) -> ()  [unwired: 2 in, 2 out]
      }
    }
  }
